vi "WHD_VEten_0.1.1_WS_BIDIR.vi"() -> ()   [LabVIEW 2015]
uses:
  <vilib>/NI_Real-Time Target Support.lvlib
  <vilib>/rvi/interface/nirviReadWriteControl/nirviReadWriteControl.xnode
  <vilib>/rvi/interface/nirviMethod/nirviMethod.xnode
  <vilib>/rvi/interface/nirviOpenFPGA/nirviOpenFPGA.xnode
  <vilib>/rvi/interface/nirviCloseFPGA/nirviCloseFPGA.xnode
  <vilib>/userdefined/High Color/nirio_resource_hc.ctl
  <vilib>/rvi/errors/niLvFpgaMergeErrorWithErrorCode.vi
  <vilib>/Utility/file.llb/Write Delimited Spreadsheet (string).vi
  <vilib>/RTwatchdog.llb/Watchdog expiration actions.ctl
  <vilib>/nisyscfg/nisyscfg.lvlib
  AURA_Wheel/Json2Labv.lvlib
  AURA_Wheel/AuraWheelAPI/AuraWheel.lvlib
  <vilib>/rvi/errors/niLvFpgaAdjustHostInterfaceError.vi
  NiFpgaLv.dll
  <vilib>/Utility/error.llb/Error Cluster From Error Code.vi
  <vilib>/LabVIEW Targets/FPGA/cRIO/shared/nicrio_ModuleControls/nicrio_cRIO-9234_DataRatesRing2.ctl
  <vilib>/FPGAPlugInAG/cRIO-9031/niLvFpga_Run_cRIO-9031.vi
  <vilib>/FPGAPlugInAG/cRIO-9031/niLvFpga_Reset_cRIO-9031.vi
  FPGA Bitfiles/W&RDArabia_FPGATarget_FPGA8a2wsBIdirec_yJvL9yuTbZw.lvbitx
  <vilib>/FPGAPlugInAG/cRIO-9031/niLvFpga_Open_cRIO-9031.vi
  <vilib>/FPGAPlugInAG/cRIO-9031/niLvFpga_ConfigureFifo_cRIO-9031.vi
  <vilib>/FPGAPlugInAG/cRIO-9031/niLvFpga_StartFifo_cRIO-9031.vi
  <vilib>/FPGAPlugInAG/cRIO-9031/niLvFpga_ReadFifo_cRIO-9031.vi
  <vilib>/FPGAPlugInAG/cRIO-9031/niLvFpga_StopFifo_cRIO-9031.vi
  <vilib>/FPGAPlugInAG/cRIO-9031/niLvFpga_Close_cRIO-9031.vi
panel:
  in  "Digital?":bool=TRUE
  out "Direction 0?":bool
  out "Boton Adquirir?":bool
  out "Wheel detected2?":bool=TRUE
  out "Wheel detected1?":bool=TRUE
  in  "Timeout ruedas":dbl
  in  "Borrar archivos\nadquisicion con error":bool
  in  "Able watchdog?":bool
  in  "Reset watchdog?":bool
  in  "Leer config RFID NEM":bool
  in  "bytes to read":i32
  in  "DeviceAddress":u8
  in  "timeout ms (60000)":i32
  in  "Max archivos":u32=2
  in  "Bytes libre despues de borrar":u32=2
  in  "Bytes min libre":u32=2
  in  "Nº de acelerómetros":i32
  in  "Nº inductivos":i32
  in  "Offset_rueda WS 1":fxp<+/-,24,-4>=0.004999998956918716 format="%.27g"
  out "TAGs_AURAwheel":string[][](array[string])
  out "Plataformas?":bool
  out "Nº Ejes":i32[](array[numeric])
  out "Nº UTs":i32
  out "it-read-LR6":i32[](array[numeric])
  out "it-LR6":i32
  out "RFID_LR6_Error":errorcluster
  out "Series_flota":string[](array[string])
  out "Tabla_flota":string[][](array[string])
  out "Puntos medios de las ventanas":dbl[][](array[numeric])
  out "configuration file path":path=path "c:/Parametros.cfg"
  in  "IP synchr":string
  out "data":cluster{"status":string}
  out "confRFID":path=path "c:/RFID/TAGS.csv"
  out "TAGS leidos":path=path "c:/RFID/TAGS.csv"
  in  "Use Aura?":bool
  in  "Parametros AuraWheel":string[](array[string])
  in  "Parámetros acelerómetros":dbl[](array[numeric])
  in  "Acquisition time":dbl=10.0
  in  "Acquire":bool
  out "Fin":bool
  out "Contador":i32=1
  out "Path TEST":path=path "c:/TEST"
  out "Fallo fotocelula":bool
  out "Path_Borrar":path=path "c:/Trenes"
  out "Longitud de la unidad":dbl
  out "Aviso no detección":string
  out "Time to Acquire Block (ms)":i32
  out "Distancia de acelerómetros":dbl[](array[numeric])
  out "Block Size":u32
  out "Distancias generales":dbl[](array[numeric])
  in  "Reset del controlador":bool
  in  "Configuración":bool
  in  "Parar la aplicación":bool
  out "RFID":bool=TRUE
  out "date/time string":string
  out "Timeout ruedas":bool
  out "Tiempo":dbl
  out "Inicio pasada":timestamp
  out "Ultimo TEST":timestamp
  out "Power Supply":bool=TRUE
  out "Status":string
  out "RFID_ID":refnum<k5>
  out "DC OK":string
  out "Aviso temperatura":string
  in  "Tab Control":T1(tab)=enum."Parameters"
  out "V (m/s)":dbl
  out "Temperature (ºC)":dbl
  out "Max Wheel RMS":dbl[][](array[numeric])
  out "result":bool
  out "TAGs":string[](array[string])
  out "Parar":bool
  out "TAGs LR6":string[](array[string])
  out "TAGs HEX":string[](array[string])
  out "Digital wheels":sgl[](graph)
  out "Current Wheel sensor":sgl[][](graph)
  out "File Name":path[](array[path])
  out "Train pass time (s)":dbl
  out "Acquisition extra time (s)":dbl
  out "Detected axles":i32
  out "Buffer Underflow":bool
  out "Buffer Overflow":bool
  out "Hard drive status (bytes)":i64
  out "created path":path
  out "Nº Wheel 1":i32
  out "Nº Wheel 2":i32
  out "Train axles":i32
  out "Valid \nfile?":bool
  in  "AURA wheel test":bool
  out "T fuera rango":bool
  in  "Frecuency rate (Hz)":dbl=25600.0
  in  "Samples per channel FIFO":u32=5000
  in  "Extra time detection (s)":dbl=1.0
  in  "dt RMS":dbl=256.0
  in  "Frecuency rate and CRIO module":T2=2 items=["51.200 kS/s (NI 9234)"=1, "25.600 kS/s (NI 9234)"=2, "17.067 kS/s (NI 9234)"=3, "12.800 kS/s (NI 9234)"=4, "10.240 kS/s (NI 9234)"=5, "8.533 kS/s (NI 9234)"=6, "7.314 kS/s (NI 9234)"=7, "6.400 kS/s (NI 9234)"=8, "5.689 kS/s (NI 9234)"=9, "5.120 kS/s (NI 9234)"=10, "4.654 kS/s (NI 9234)"=11, "4.267 kS/s (NI 9234)"=12, "3.938 kS/s (NI 9234)"=13, "3.657 kS/s (NI 9234)"=14, "3.413 kS/s (NI 9234)"=15, "3.200 kS/s (NI 9234)"=16, "3.012 kS/s (NI 9234)"=17, "2.845 kS/s (NI 9234)"=18, "2.695 kS/s (NI 9234)"=19, "2.560 kS/s (NI 9234)"=20, "2.438 kS/s (NI 9234)"=21, "2.328 kS/s (NI 9234)"=22, "2.226 kS/s (NI 9234)"=23, "2.133 kS/s (NI 9234)"=24, "2.048 kS/s (NI 9234)"=25, "1.969 kS/s (NI 9234)"=26, "1.896 kS/s (NI 9234)"=27, "1.829 kS/s (NI 9234)"=28, "1.765 kS/s (NI 9234)"=29, "1.707 kS/s (NI 9234)"=30, "1.652 kS/s (NI 9234)"=31]
  in  "RFID Port":u16=2189
  in  "RFID IP":string="192.168.106.99"
  in  "Offset_rueda WS 2":fxp<+/-,24,-4>=0.004999998956918716 format="%.27g"
  in  "Count(mSec)":u32=2
  in  "LR6 IP address":string="192.168.106.94"
  in  "Port LR6":u16=2001
  in  "RFID NEM on?":bool
  in  "RFID LR6 on?":bool
  in  "Zero channel WS1?":bool
  in  "Zero channel WS2?":bool
  out "Parameters":bool=TRUE
  out "Distances of the system":bool=TRUE
  out "RFID Error":errorcluster
  out "FPGA error":errorcluster
  out "Write/read error":errorcluster
  out "Units and axles":bool=TRUE
  out "RFID":bool=TRUE
  out "AURA error":errorcluster
  out "Response headers":string
  out "Numeric 3":i32
  out "Loop":i32
  out "Watchdog config":T3={"reset system"=FALSE, "restart LabVIEW Runtime"=FALSE, "occurrence"=FALSE, "trigger protocol"=enum."active high", "trigger line"=enum."none", "disable watchdog on VI exit"=TRUE}
  # "Last train detected"
  # "Error!!"
  # "Memory status"
  # "Samples parameters"
  # "Acquisition parameters"
  # "Other parameters"
  # "Configuration data load"
  # "Errores!!"
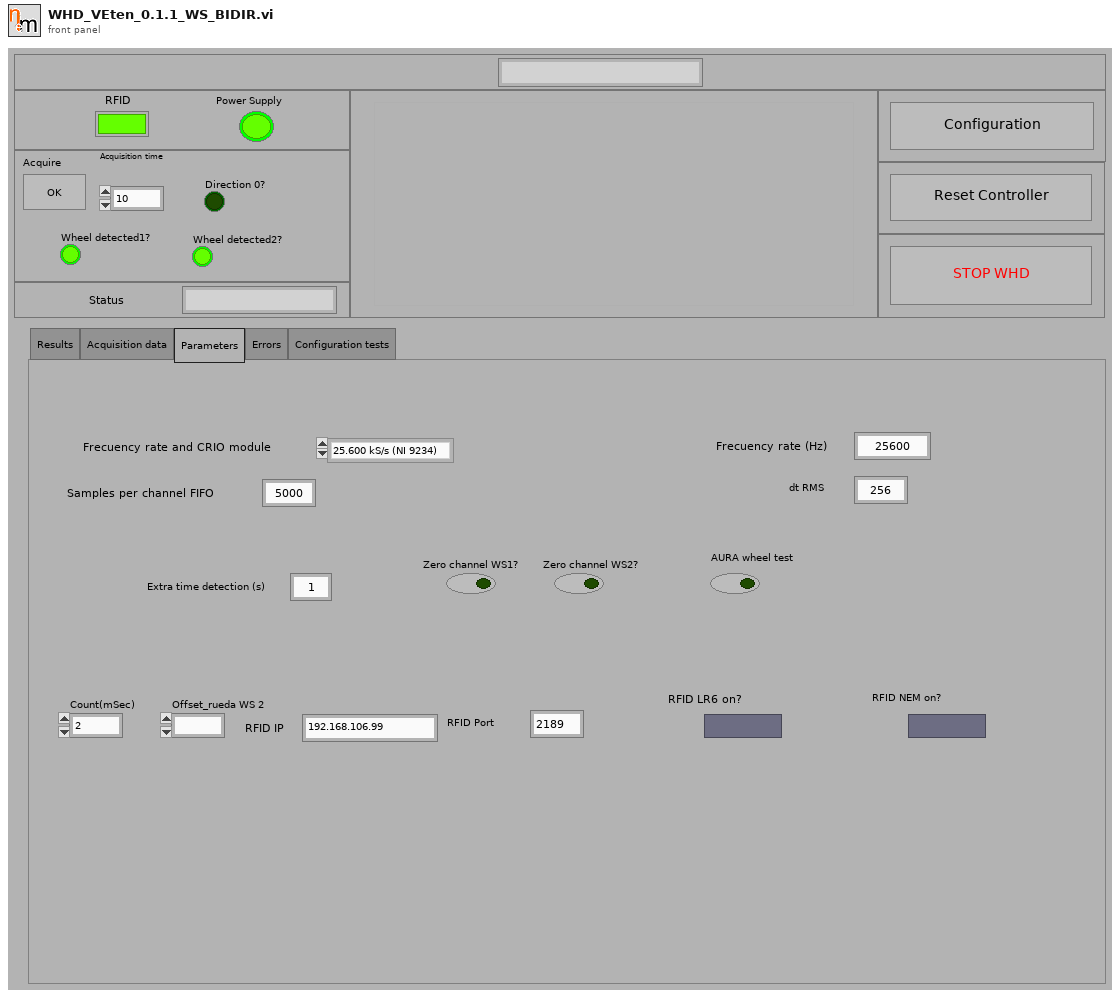
[diagram p1: front panel]
types:
  T1 = enum32{"Results", "Acquisition data", "Parameters", "Errors", "Configuration tests"}
  T2 = typedef "nicrio_cRIO-9234_DataRatesRing2.ctl" = u8
  T3 = typedef "Watchdog expiration actions.ctl" = cluster{"reset system":bool, "restart LabVIEW Runtime":bool, "occurrence":bool, "trigger protocol":enum16{"active high", "active low", "open collector"}, "trigger line":enum16{"none", "line 0", "line 1", "line 2", "line 3", "line 4", "line 5", "line 6", "line 7", "SMB line 0"}, "disable watchdog on VI exit":bool}
  T4 = typedef "nirio_resource_hc.ctl" = tag
  T5 = enum16{"Standard", "Buffered", "CRLF", "Immediate"}
  T6 = enum16{"open", "replace", "create", "open or create", "replace or create", "replace or create with confirmation"}
  T7 = enum16{"big-endian, network order", "native, host order", "little-endian"}
  T8 = cluster{"error IO":errorcluster, bool[], u32[], string[], dbl[]}
  T9 = cluster{"g_ts":dbl, "p_sp":dbl, "p_tp":dbl, "p_tg":cluster{"tg_n":dbl, "tg_t":string}[], "p_ax":cluster{"ax_n":dbl, "ax_sp":dbl, "ax_wh":cluster{"wh_p":dbl, "wh_a1":dbl, "wh_a2":dbl, "wh_a3":dbl, "wh_a4":dbl}[]}[]}
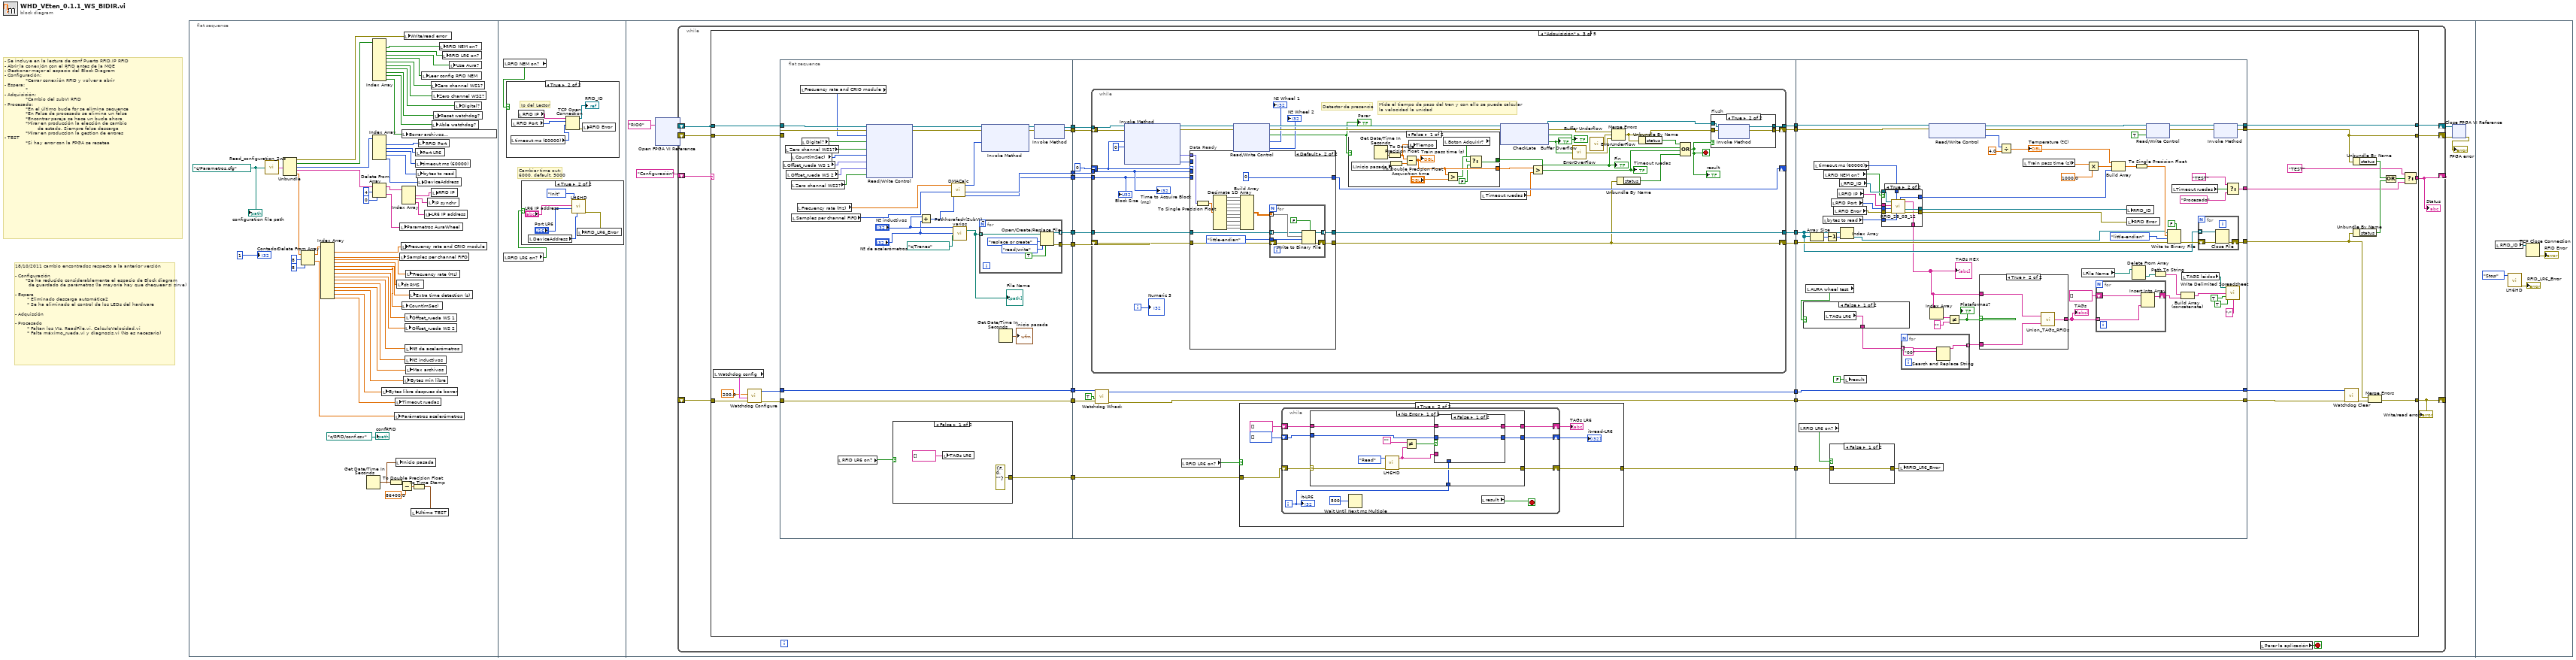
[diagram p0: block diagram]
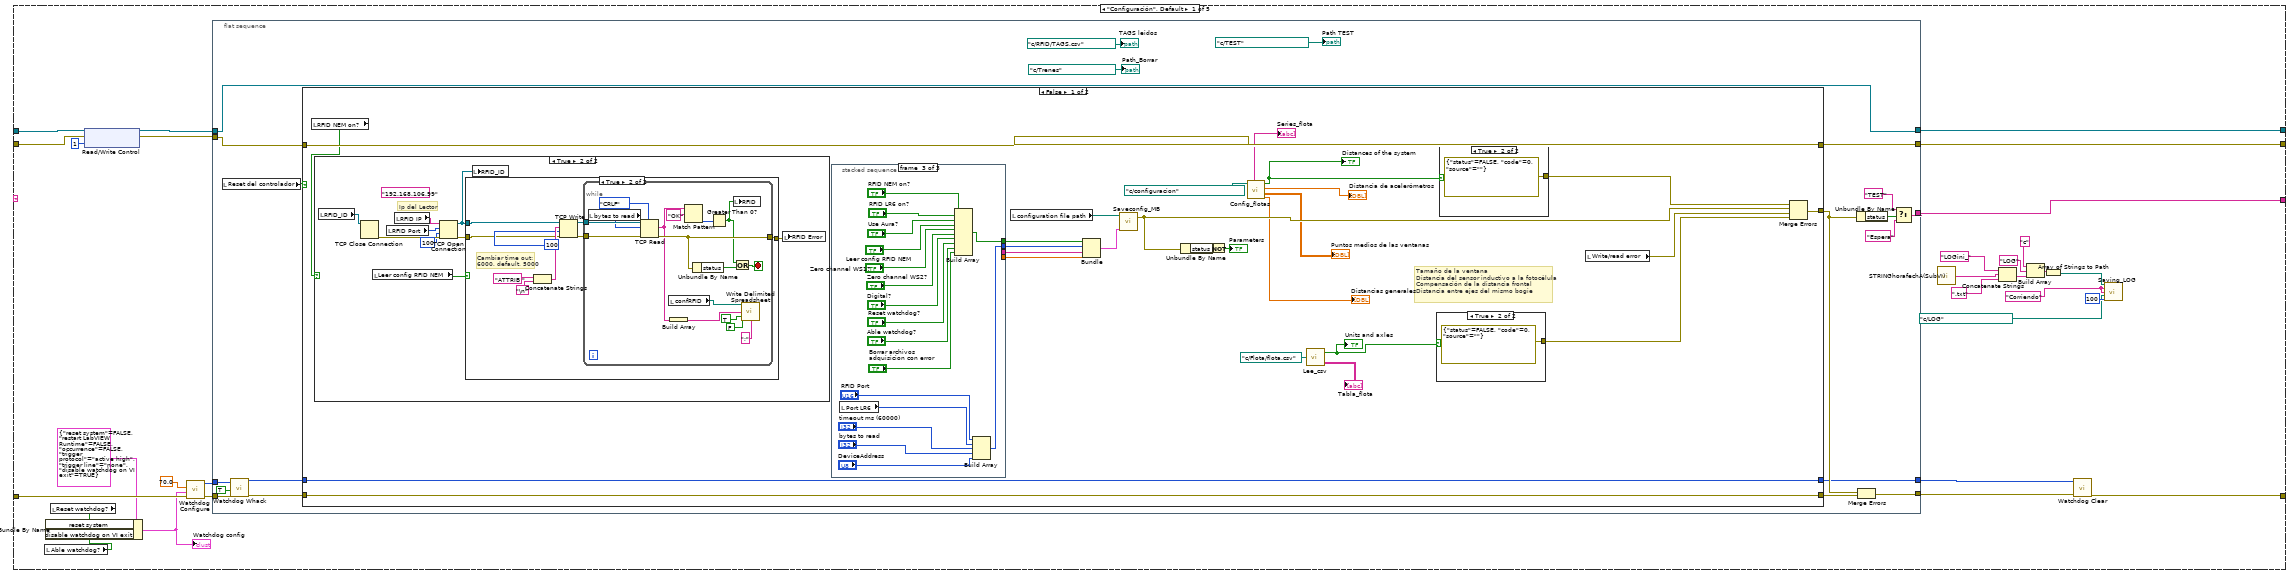
[diagram p4: hidden frame]
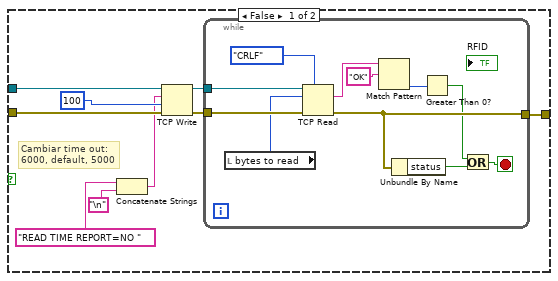
[diagram p6: hidden frame]
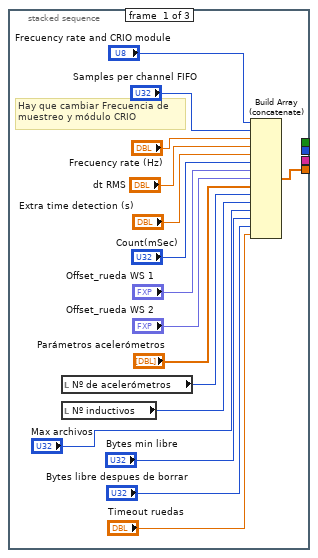
[diagram p7: hidden frame]
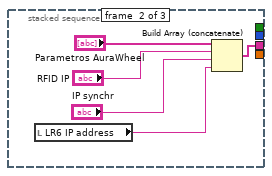
[diagram p8: hidden frame]
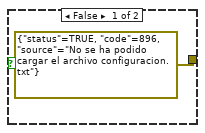
[diagram p9: hidden frame]
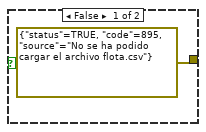
[diagram p10: hidden frame]
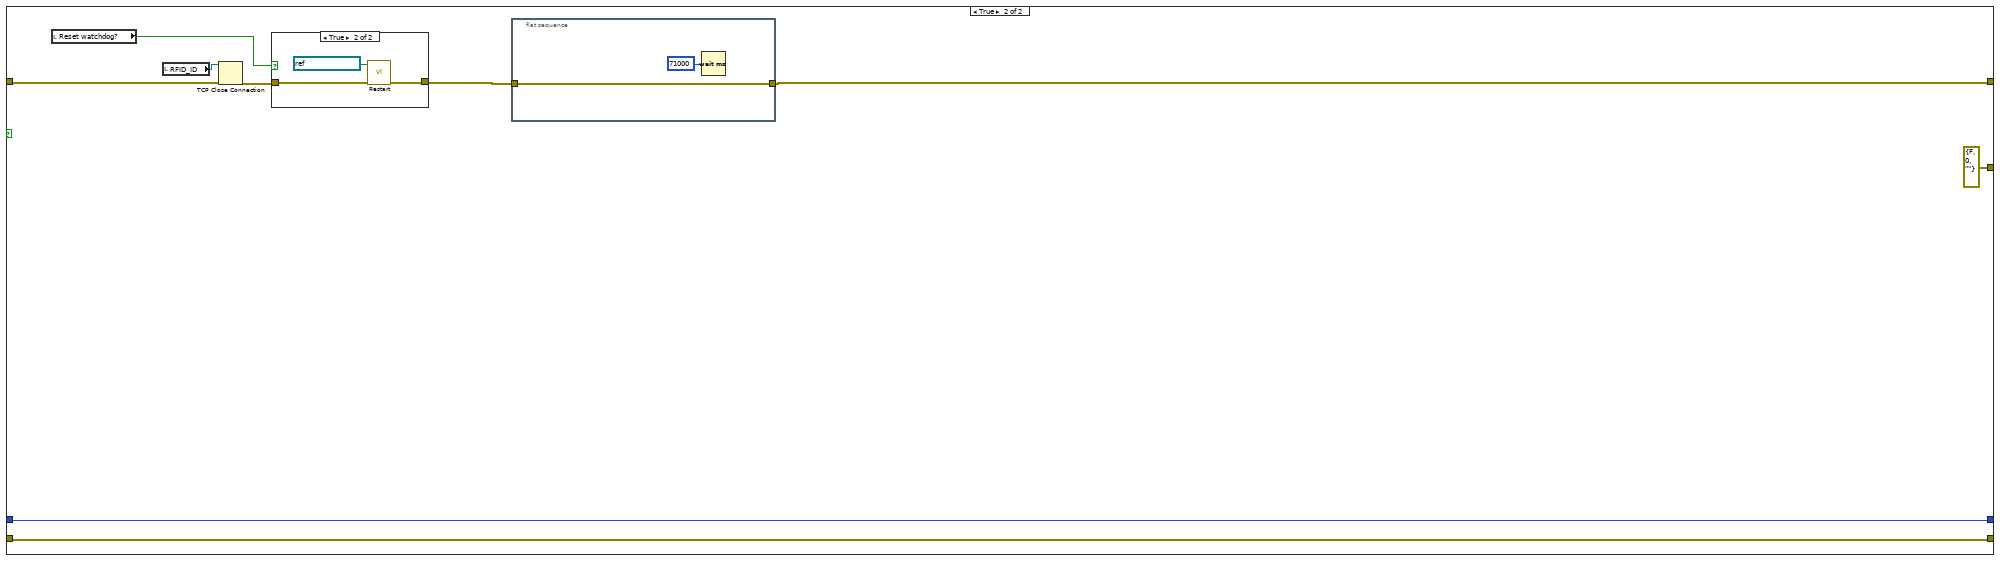
[diagram p11: hidden frame]
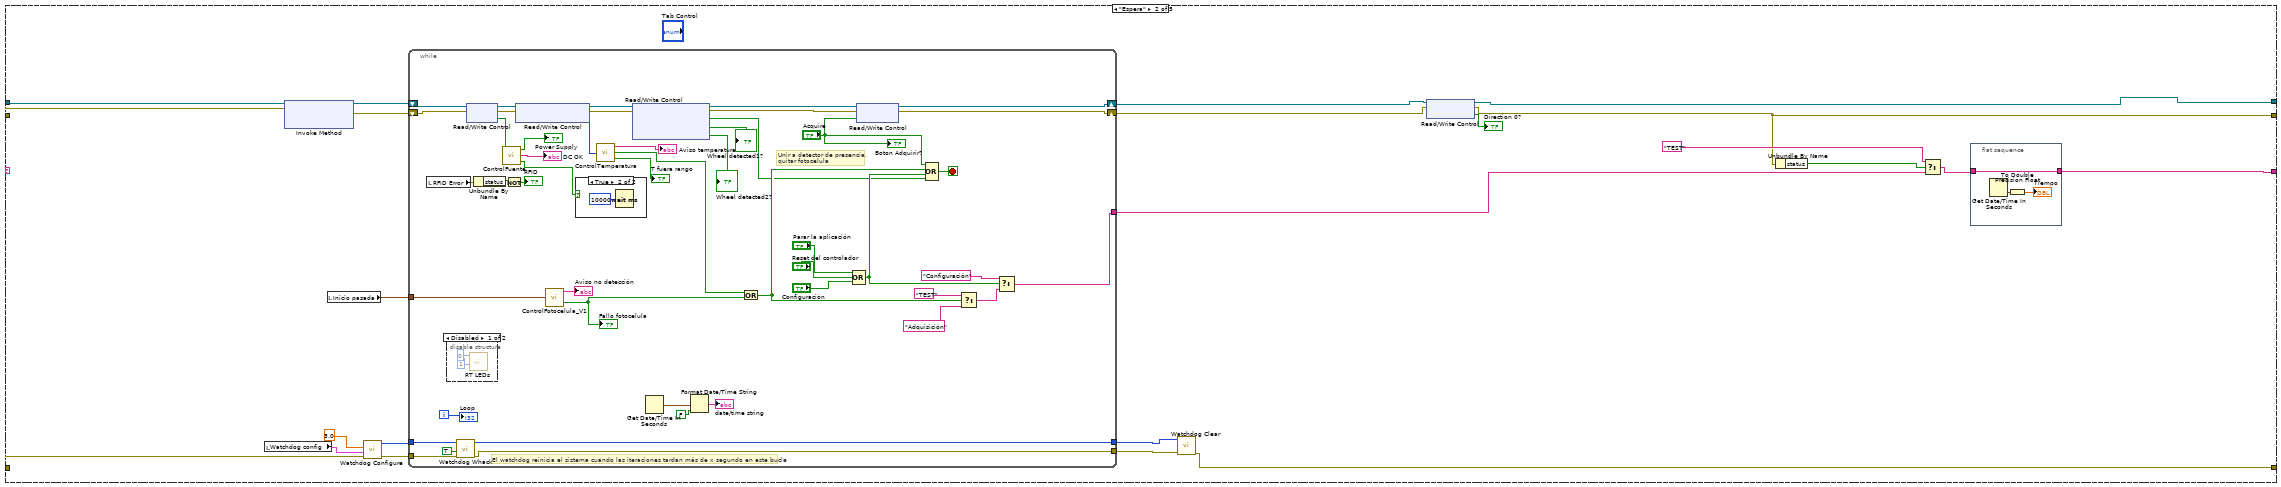
[diagram p13: hidden frame]
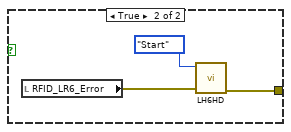
[diagram p16: hidden frame]
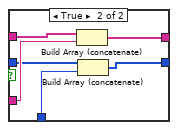
[diagram p18: hidden frame]
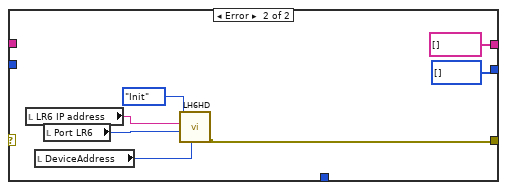
[diagram p19: hidden frame]
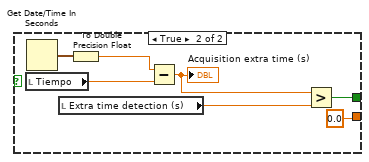
[diagram p20: hidden frame]
diagram:
  # "18/10/2011 cambio encontrados respecto a la anterior versión\n\n- Configuración\n       *Se ha reducido considerablemente el espacio de Block diagram\n         de guardado de parámetros (la mayoría hay que chequear si sirve)\n\n- Espera\n        * Eliminado descarga automática2\n        * Se ha eliminado el control de los LEDs del hardware\n       \n- Adquisción\n\n- Procesado\n        * Faltan los VIs, ReadFile.vi, CalculoVelocidad.vi\n        * Falta máximo_rueda.vi y diagnosis.vi (No es necesario)"
  # "- Se incluye en la lectura de conf Puerto RFID,IP RFID\n- Abrir la conexión con el RFID antes de la MQE\n- Gestionar mejor el espacio del Block Diagram\n- Configuración:\n              *Cerrar conexión RFID y volver a abrir\n- Espera:\n              *\n- Adquisición:\n              *Cambio del subVI RFID\n- Procesado:\n              *En el último bucle for se elimina sequence\n              *En False de procesado se elimina un false\n              *Encontrar pareja se hace un bucle ahora\n              *Mirar en producción la elección de cambio\n                      de estado. Siempre false descarga \n              *Mirar en produccion la gestion de errores\n- TEST\n              *Si hay error con la FPGA se resetea"
  n1 = flat-sequence {
    frame #0 {
      w38 = path "c:/Parametros.cfg" ("configuration file path")
      n2 = call "Read_configuration_2ws.vi"("configuration file path"=w38) -> ("output cluster"=w37:T8)
      n3 = Unbundle(w37) -> ("error IO"=w42:errorcluster, w41:bool[], w40:u32[], w29:string[], w35:dbl[])
      n4 = Delete From Array(array=w35, length=8, index=8) -> (deleted portion=w31:dbl[], array with subset deleted=w34:dbl[])
      n5 = Index Array(array=w34) -> (element #1=w49:dbl, element #2=w48:dbl, element #3=w47:dbl, element #4=w46:dbl, element #5=w45:dbl, element #6=w19:dbl, element #7=w18:dbl, element #8=w1:dbl, element #9=w17:dbl, element #10=w16:dbl, element #11=w15:dbl, element #12=w14:dbl, element #13=w13:dbl, element #14=w2:dbl)  [unwired: 14 in]
      n6 = Get Date/Time In Seconds() -> (seconds since 1Jan1904=w51:timestamp)
      n7 = Index Array(array=w41) -> (element #1=w44:bool, element #2=w43:bool, element #3=w30:bool, element #4=w9:bool, element #5=w8:bool, element #6=w7:bool, element #7=w6:bool, element #8=w5:bool, element #9=w4:bool, element #10=w3:bool)  [unwired: 10 in]
      n8 = Index Array(array=w40) -> (element #1=w36:u32, element #2=w20:u32, element #3=w12:u32, element #4=w11:u32, element #5=w10:u32)  [unwired: 5 in]
      n9 = Delete From Array(array=w29, length=4, index=0) -> (deleted portion=w23:string[], array with subset deleted=w28:string[])
      n10 = local write "Bytes libre despues de borrar"(w13) -> ()
      n11 = To Double Precision Float(number=w51) -> (double precision float=w53:dbl)
      n12 = local write "Parámetros acelerómetros"(w31) -> ()
      n13 = local write "Timeout ruedas"(w2) -> ()
      n14 = local write "Inicio pasada"(w51) -> ()
      n15 = local write "dt RMS"(w46) -> ()
      n16 = local write "Samples per channel FIFO"(w48) -> ()
      n17 = local write "Parametros AuraWheel"(w23) -> ()
      n18 = Subtract(x=w53, y=86400.0) -> (x-y=w52:dbl)
      n19 = local write "Frecuency rate and CRIO module"(w49) -> ()
      n20 = local write "Borrar archivos\nadquisicion con error"(w3) -> ()
      n21 = Index Array(array=w28) -> (element #1=w22:string, element #2=w24:string, element #3=w21:string)  [unwired: 3 in]
      n22 = local write "Count(mSec)"(w19) -> ()
      n23 = local write "Bytes min libre"(w14) -> ()
      n24 = local write "Write/read error"(w42) -> ()
      n25 = local write "Offset_rueda WS 2"(w1) -> ()
      n26 = local write "Offset_rueda WS 1"(w18) -> ()
      n27 = local write "Nº de acelerómetros"(w17) -> ()
      n28 = local write "Nº inductivos"(w16) -> ()
      n29 = local write "Frecuency rate (Hz)"(w47) -> ()
      n30 = local write "Max archivos"(w15) -> ()
      n31 = local write "Extra time detection (s)"(w45) -> ()
      n32 = To Time Stamp(1:w52) -> (0:w50:timestamp)
      n33 = local write "Ultimo TEST"(w50) -> ()
      n34 = local write "Port LR6"(w20) -> ()
      n35 = local write "timeout ms (60000)"(w12) -> ()
      n36 = local write "bytes to read"(w11) -> ()
      n37 = local write "DeviceAddress"(w10) -> ()
      n38 = local write "RFID Port"(w36) -> ()
      n39 = local write "Leer config RFID NEM"(w9) -> ()
      n40 = local write "LR6 IP address"(w21) -> ()
      n41 = local write "IP synchr"(w24) -> ()
      n42 = local write "Zero channel WS1?"(w8) -> ()
      n43 = local write "RFID IP"(w22) -> ()
      n44 = local write "Able watchdog?"(w4) -> ()
      n45 = local write "Zero channel WS2?"(w7) -> ()
      n46 = local write "Reset watchdog?"(w5) -> ()
      n47 = local write "RFID NEM on?"(w44) -> ()
      n48 = local write "RFID LR6 on?"(w43) -> ()
      n49 = local write "Use Aura?"(w30) -> ()
      n50 = local write "Digital?"(w6) -> ()
      "Contador" <- 1
      "confRFID" <- path "c:/RFID/conf.csv" ("file path (use dialog)")
      "configuration file path" <- w38
    }
    frame #1 {
      # "Cambiar time out:\n6000, default, 5000"
      n51 = local read "RFID NEM on?"() -> (w56:bool)
      n52 = local read "RFID LR6 on?"() -> (w55:bool)
      n53 = case shown="True" w56 {
        frame False {
        }
        frame True {
          # "Ip del Lector"
          n54 = local read "timeout ms (60000)"() -> (w62:i32)
          n55 = local read "RFID Port"() -> (w64:u16)
          n56 = local read "RFID IP"() -> (w65:string)
          n57 = TCP Open Connection(address=w65, remote port or service name=w64, timeout ms (60000)=w62) -> (connection ID=→"RFID_ID":refnum<k5>, error out=w63:errorcluster)  [unwired: 1 in, 1 out]
          n58 = local write "RFID Error"(w63) -> ()
        }
      }
      n59 = case shown="True" w55 {
        frame False {
        }
        frame True {
          n60 = local read "DeviceAddress"() -> (w57:u8)
          n61 = call "LH6HD.vi"("DeviceAddress"=w57, "Reader Port"="Port LR6", "IP Address"="LR6 IP address", "Action"=enum16{"Init", "Start", "Read", "Stop", "Exit"}."Init") -> ("error out"=w61:errorcluster)  [unwired: 6 in, 1 out]
          n62 = local write "RFID_LR6_Error"(w61) -> ()
        }
      }
    }
    frame #2 {
      n63 = xnode "Open FPGA VI Reference"("resource name"=T4 "RIO0") -> ("FPGA VI Reference Out"=w73:refnum<k20>, "error out"=w72:errorcluster)  [unwired: 1 in]
      n64 = while {
        shift-right: [w77] -> _
        shift-left: "Configuración" -> [w82]
        shift-right: [w75] -> w69
        shift-left: w73 -> [w81]
        shift-right: [w74] -> w68
        shift-left: w72 -> [w80]
        shift-right: [w79] -> _
        shift-left: _ -> [w78]
        stop <- w76 stop-if-true
        n65 = case shown="\"Adquisición\"" w82 {
          tunnel: [w111 w283 w360 w695 w942] -> w77
          tunnel: [w110 w271 w374 w703 w941] -> w75
          tunnel: [w112 w270 w375 w690 w939] -> w74
          tunnel: w81 -> [w99 w288 w382 w703 w941]
          tunnel: w80 -> [w97 w286 w381 w690 w940]
          tunnel: [w103 w277 w372 w693 w929] -> w79
          tunnel: w78 -> [w109 w282 w356 w689 w934]
          frame "Configuración", Default {
            w83 = "Corriendo" ("Report")
            n66 = local read "Able watchdog?"() -> (w94:bool)
            n67 = local read "Reset watchdog?"() -> (w101:bool)
            n68 = Bundle By Name(cluster=T3 {"reset system"=FALSE, "restart LabVIEW Runtime"=FALSE, "occurrence"=FALSE, "trigger protocol"=enum."active high", "trigger line"=enum."none", "disable watchdog on VI exit"=TRUE} ("expiration actions"), "reset system"=w101, "disable watchdog on VI exit"=w94) -> (w100:T3)
            "Watchdog config" <- w100
            n69 = xnode "Read/Write Control"("FPGA VI Reference In"=w99, "error in"=w97, "Cycles to Filter"=u16 1) -> ("FPGA VI Reference Out"=w98:refnum<k20>, "error out"=w96:errorcluster)
            n70 = call <vilib>:"Watchdog Configure.vi"("error in (no error)"=w109, "expiration actions"=w100, "timeout (1 sec)"=70.0) -> ("error out"=w106:errorcluster, "watchdogID"=w107:u64)  [unwired: 1 in, 2 out]
            n71 = flat-sequence {
              tunnel: [w123] -> w112
              tunnel: [w131] -> w111
              tunnel: w98 -> [w124]
              tunnel: [w124] -> w110
              tunnel: [w126] -> w104
              tunnel: w96 -> [w121]
              tunnel: w107 -> [w119]
              tunnel: w106 -> [w118]
              tunnel: [w116] -> w105
              frame #0 {
                n72 = local read "Reset del controlador"() -> (w120:bool)
                n73 = call <vilib>:"Watchdog Whack.vi"("error in (no error)"=w118, "reset watchdog after expire? (F)"=TRUE, "watchdogID in"=w119) -> ("error out"=w114:errorcluster, "watchdogID out"=w115:u64)  [unwired: 2 in, 1 out]
                n74 = case shown="False" w120 {
                  tunnel: w121 -> [w158 w261]
                  tunnel: [w158 w260] -> w123
                  tunnel: [w144 errorcluster {"status"=FALSE, "code"=0, "source"=""} ("error IO")] -> w122
                  tunnel: [w136 w259] -> w116
                  tunnel: w115 -> [w136 w259]
                  tunnel: w114 -> [w135 w258]
                  tunnel: [w135 w258] -> w113
                  frame False {
                    # "Tamaño de la ventana\nDistancia del sensor inductivo a la fotocélula\nCompensación de la distancia frontal\nDistancia entre ejes del mismo bogie"
                    n75 = local read "RFID NEM on?"() -> (w134:bool)
                    n76 = case shown="True" w134 {
                      frame False {
                      }
                      frame True {
                        (unwired) "192.168.106.99" ("address")
                        # "Ip del Lector"
                        n77 = local read "RFID_ID"() -> (w166:refnum<k5>)
                        n78 = TCP Close Connection(connection ID=w166) -> (error out=w167:errorcluster)  [unwired: 2 in, 1 out]
                        n79 = local read "Leer config RFID NEM"() -> (w159:bool)
                        n80 = local read "RFID Port"() -> (w164:u16)
                        n81 = local read "RFID IP"() -> (w163:string)
                        n82 = TCP Open Connection(address=w163, remote port or service name=w164, timeout ms (60000)=100, error in (no error)=w167) -> (connection ID=w165:refnum<k5>, error out=w160:errorcluster)  [unwired: 1 out]
                        n83 = case shown="True" w159 {
                          tunnel: w165 -> [w176 w190]
                          tunnel: [w174 w188] -> w161
                          tunnel: w160 -> [w171 w189]
                          frame False {
                            # "Cambiar time out:\n6000, default, 5000"
                            n84 = Concatenate Strings("READ TIME REPORT=NO " ("data in"), "\n") -> (w168:string)
                            n85 = TCP Write(connection ID=w176, data in=w168, error in (no error)=w171, 9:100 ("timeout ms (25000)")) -> (connection ID out=w172:refnum<k5>, error out=w173:errorcluster)  [unwired: 1 out]
                            n86 = while {
                              tunnel: w173 -> [w186]
                              tunnel: w172 -> [w185]
                              tunnel: [w184] -> w174
                              stop <- w181 stop-if-true
                              n87 = local read "bytes to read"() -> (w177:i32)
                              n88 = TCP Read(connection ID=w185, bytes to read=w177, error in (no error)=w186, 7:T5."CRLF" ("mode (standard)")) -> (data out=w179:string, error out=w184:errorcluster)  [unwired: 1 in, 1 out]
                              n89 = Match Pattern(string=w179, regular expression="OK") -> (offset past match=w182:i32)  [unwired: 4 out]
                              n90 = Unbundle By Name(w184) -> ("status"=w180:bool)
                              n91 = Greater Than 0?(x=w182) -> (x > 0?=w178:bool)
                              n92 = Or(x=w178, y=w180) -> (x .or. y?=w181:bool)
                            }
                          }
                          frame True {
                            # "Cambiar time out:\n6000, default, 5000"
                            n93 = Concatenate Strings("ATTRIB " ("data in"), "\n") -> (w196:string)
                            n94 = TCP Write(connection ID=w190, data in=w196, error in (no error)=w189, 9:100 ("timeout ms (25000)")) -> (connection ID out=w193:refnum<k5>, error out=w192:errorcluster)  [unwired: 1 out]
                            n95 = while {
                              tunnel: w192 -> [w211]
                              tunnel: w193 -> [w210]
                              tunnel: [w209] -> w188
                              stop <- w206 stop-if-true
                              n96 = local read "bytes to read"() -> (w198:i32)
                              n97 = TCP Read(connection ID=w210, bytes to read=w198, error in (no error)=w211, 7:T5."CRLF" ("mode (standard)")) -> (data out=w201:string, error out=w209:errorcluster)  [unwired: 1 in, 1 out]
                              n98 = local read "confRFID"() -> (w200:path)
                              n99 = Build Array(w201) -> (w199:string[])
                              n100 = Match Pattern(string=w201, regular expression="OK") -> (offset past match=w207:i32)  [unwired: 4 out]
                              n101 = Unbundle By Name(w209) -> ("status"=w205:bool)
                              n102 = Greater Than 0?(x=w207) -> (x > 0?=w197:bool)
                              n103 = local write "RFID"(w197) -> ()
                              n104 = Or(x=w197, y=w205) -> (x .or. y?=w206:bool)
                              n105 = call-poly <vilib>:"Write Delimited Spreadsheet.vi"("file path (dialog if empty)"=w200, "1D data"=w199, "append to file? (new file:F)"=FALSE ("transpose? (no:F)"), "transpose? (no:F)"=TRUE ("append to file? (new file:F)"), "delimiter (\\t)"=";" ("delimiter (\\t)")) -> ()  [unwired: 9 in, 2 out]
                            }
                          }
                        }
                        n106 = local write "RFID_ID"(w165) -> ()
                        n107 = local write "RFID Error"(w161) -> ()
                      }
                    }
                    n108 = stacked-sequence {
                      tunnel: [w224 _ _] -> w148
                      tunnel: [_ w233 _] -> w147
                      tunnel: [_ _ w247] -> w149
                      tunnel: [_ _ w246] -> w150
                      frame #0 {
                        # "Hay que cambiar Frecuencia de\nmuestreo y módulo CRIO"
                        n109 = local read "Nº de acelerómetros"() -> (w218:i32)
                        n110 = local read "Nº inductivos"() -> (w217:i32)
                        n111 = Build Array (concatenate)("Frecuency rate and CRIO module", "Samples per channel FIFO", "Frecuency rate (Hz)", "dt RMS", "Extra time detection (s)", "Count(mSec)", "Offset_rueda WS 1", "Offset_rueda WS 2", "Parámetros acelerómetros", w218, w217, "Max archivos", "Bytes min libre", "Bytes libre despues de borrar", "Timeout ruedas") -> (w224:dbl[])
                      }
                      frame #1 {
                        n112 = local read "LR6 IP address"() -> (w229:string)
                        n113 = Build Array (concatenate)("Parametros AuraWheel", "RFID IP", "IP synchr", w229) -> (w233:string[])
                      }
                      frame #2 {
                        n114 = local read "Port LR6"() -> (w243:u16)
                        n115 = Build Array("RFID NEM on?", "RFID LR6 on?", "Use Aura?", "Leer config RFID NEM", "Zero channel WS1?", "Zero channel WS2?", "Digital?", "Reset watchdog?", "Able watchdog?", "Borrar archivos\nadquisicion con error") -> (w246:bool[])
                        n116 = Build Array("RFID Port", w243, "timeout ms (60000)", "bytes to read", "DeviceAddress") -> (w247:i32[])
                      }
                    }
                    n117 = local read "configuration file path"() -> (w145:path)
                    n118 = Bundle(w150, w149, w147, w148) -> (w146:cluster{bool[], i32[], string[], dbl[]})  [unwired: 1 in]
                    n119 = call "Saveconfig_MB.vi"("configuration file path"=w145, "Configuracion"=w146) -> ("error out"=w153:errorcluster)  [unwired: 4 in]
                    n120 = Unbundle By Name(w153) -> ("status"=w154:bool)
                    n121 = Not(x=w154) -> (.not. x?=→"Parameters":bool)
                    n122 = call "Config_flotas.vi"("file path (dialog if empty)"=path "c:/configuracion") -> ("Distancias generales"=→"Distancias generales":dbl[], "Puntos medios de las ventanas"=→"Puntos medios de las ventanas":dbl[][], "Distancia de acelerómetros"=→"Distancia de acelerómetros":dbl[], "Distacias y medidas de dispositivos"=w143:bool, "Series_flota"=→"Series_flota":string[])  [unwired: 3 in]
                    "Distances of the system" <- w143
                    n123 = call "Lee_csv.vi"("Path"=path "c:/Flota/flota.csv") -> ("Tabla_flota"=→"Tabla_flota":string[][], "Lectura_OK?"=w140:bool)
                    "Units and axles" <- w140
                    n124 = case shown="True" w140 {
                      tunnel: [errorcluster {"status"=TRUE, "code"=895, "source"="No se ha podido cargar el archivo flota.csv"} ("error out") errorcluster {"status"=FALSE, "code"=0, "source"=""} ("error out")] -> w151
                      frame False {
                      }
                      frame True {
                      }
                    }
                    n125 = case shown="True" w143 {
                      tunnel: [errorcluster {"status"=TRUE, "code"=896, "source"="No se ha podido cargar el archivo configuracion.txt"} ("error out") errorcluster {"status"=FALSE, "code"=0, "source"=""} ("error out")] -> w156
                      frame False {
                      }
                      frame True {
                      }
                    }
                    n126 = local read "Write/read error"() -> (w152:errorcluster)
                    n127 = Merge Errors(w156, w153, w152, w151) -> (w144:errorcluster)
                  }
                  frame True {
                    n128 = local read "Reset watchdog?"() -> (w255:bool)
                    n129 = local read "RFID_ID"() -> (w263:refnum<k5>)
                    n130 = TCP Close Connection(connection ID=w263, error in (no error)=w261) -> (error out=w257:errorcluster)  [unwired: 2 out]
                    n131 = case shown="True" w255 {
                      tunnel: w257 -> [w264 w267]
                      tunnel: [w264 w266] -> w256
                      frame False {
                      }
                      frame True {
                        n132 = call <vilib>:"Restart.vi"("error in (no error)"=w267, "Session in"=refnum<k21> "localhost") -> ("error out"=w266:errorcluster)  [unwired: 7 in, 2 out]
                      }
                    }
                    n133 = flat-sequence {
                      tunnel: [w269] -> w260
                      tunnel: w256 -> [w269]
                      frame #0 {
                        n134 = Wait (ms)(milliseconds to wait=u32 71000) -> ()  [unwired: 1 out]
                      }
                    }
                  }
                }
                n135 = Unbundle By Name(w122) -> ("status"=w132:bool)
                n136 = Merge Errors(w122, w113) -> (w126:errorcluster)
                n137 = Select(t="TEST", s=w132, f="Espera") -> (s? t:f=w131:string)
                "Path_Borrar" <- path "c:/Trenes" ("file path (use dialog)")
                "Path TEST" <- path "c:/TEST" ("file path (use dialog)")
                "TAGS leidos" <- path "c:/RFID/TAGS.csv" ("file path (use dialog)")
              }
            }
            n138 = call "STRINGhorafechA(SubVI).vi"() -> ("STRINGhora_fecha"=w91:string)
            n139 = Concatenate Strings("LOGini_" ("string"), w91, ".txt" ("string")) -> (w93:string)
            n140 = Build Array("c", "LOG" ("element"), w93) -> (w90:string[])
            n141 = Array of Strings to Path(0:w90) -> (2:w86:path)  [unwired: 1 out]
            n142 = call <vilib>:"Watchdog Clear.vi"("error in (no error)"=w104, "watchdogID in"=w105) -> ("error out"=w103:errorcluster)  [unwired: 5 in]
            n143 = call "Saving_LOG.vi"("Path"=w86, "Report"=w83, "Report AURA"=w83, "Path Carpeta"=path "c:/LOG" ("file path (use dialog)"), "Nº Archivos Max"=100) -> ()  [unwired: 9 in, 2 out]
          }
          frame "Espera" {
            n144 = local read "Watchdog config"() -> (w276:T3)
            n145 = xnode "Invoke Method"("FPGA VI Reference In"=w288, "error in"=w286) -> ("FPGA VI Reference Out"=w287:refnum<k20>, "error out"=w285:errorcluster)  [unwired: 1 in]
            n146 = local read "Inicio pasada"() -> (w292:timestamp)
            n147 = call <vilib>:"Watchdog Configure.vi"("error in (no error)"=w282, "expiration actions"=w276, "timeout (1 sec)"=3.0) -> ("error out"=w281:errorcluster, "watchdogID"=w280:u64)  [unwired: 1 in, 2 out]
            n148 = while {
              tunnel: [w316] -> w291
              shift-right: [w306] -> w272
              shift-left: w287 -> [w318]
              shift-right: [w305] -> w273
              shift-left: w285 -> [w317]
              tunnel: w292 -> [w321]
              tunnel: w281 -> [w303]
              tunnel: w280 -> [w304]
              tunnel: [w302] -> w279
              tunnel: [w301] -> w278
              i -> [w299]
              stop <- w343 stop-if-true
              # "Unir a detector de presencia,\nquitar fotocelula"
              # "El watchdog reinicia el sistema cuando las iteraciones tardan más de x segundo en este bucle"
              n149 = local read "RFID Error"() -> (w324:errorcluster)
              n150 = disable-structure shown="Disabled" {
                frame Disabled {
                  n151 = call <vilib>:"RT LEDs.vi"("State"=1, "LED Num"=0) -> ()  [unwired: 1 in, 5 out]
                }
                frame Enabled {
                }
              }
              n152 = call <vilib>:"Watchdog Whack.vi"("error in (no error)"=w303, "reset watchdog after expire? (F)"=TRUE, "watchdogID in"=w304) -> ("error out"=w301:errorcluster, "watchdogID out"=w302:u64)  [unwired: 2 in, 1 out]
              n153 = xnode "Read/Write Control"("FPGA VI Reference In"=w318, "error in"=w317) -> ("FPGA VI Reference Out"=w334:refnum<k20>, "error out"=w333:errorcluster, "DC OK"=w338:bool)
              n154 = Unbundle By Name(w324) -> ("status"=w322:bool)
              n155 = call "ControlFuente.vi"("DC OK 3"=w338) -> ("DC OK 2"=→"Power Supply":bool, "DC OK"=→"DC OK":string, "Boolean"=w296:bool)
              n156 = Not(x=w322) -> (.not. x?=→"RFID":bool)
              n157 = xnode "Read/Write Control"("FPGA VI Reference In"=w334, "error in"=w333) -> ("FPGA VI Reference Out"=w330:refnum<k20>, "error out"=w329:errorcluster, "Chassis Temperature"=w336:i16)
              n158 = call "ControlFotocelula_V1.vi"("Tiempo de entrada a espera"=w321) -> ("Aviso no detección"=→"Aviso no detección":string, "Boolean"=w327:bool)
              "Fallo fotocelula" <- w327
              n159 = case shown="True" w296 {
                frame False {
                }
                frame True {
                  n160 = Wait (ms)(milliseconds to wait=u32 10000) -> ()  [unwired: 1 out]
                }
              }
              n161 = call "ControlTemperatura.vi"("Chassis Temperature"=w336) -> ("Aviso temperatura"=→"Aviso temperatura":string, "Boolean"=w297:bool, "T fuera rango"=→"T fuera rango":bool)
              n162 = xnode "Read/Write Control"("FPGA VI Reference In"=w330, "error in"=w329) -> ("FPGA VI Reference Out"=w320:refnum<k20>, "error out"=w319:errorcluster, "Detector de presencia"=w311:bool, "RuedaDetectada1?"=→"Wheel detected1?":bool, "RuedaDetectada2?"=→"Wheel detected2?":bool)
              n163 = Get Date/Time In Seconds() -> (seconds since 1Jan1904=w313:timestamp)
              n164 = Format Date/Time String(seconds (now)=w313, UTC format=FALSE) -> (date/time string=→"date/time string":string)  [unwired: 1 in]
              n165 = Compound Arithmetic op=OR(w297, w327) -> (w328:bool)
              n166 = Compound Arithmetic op=OR("Parar la aplicación", "Reset del controlador", "Configuración") -> (w325:bool)
              n167 = xnode "Read/Write Control"("FPGA VI Reference In"=w320, "error in"=w319, "Fotocélula"="Acquire") -> ("FPGA VI Reference Out"=w306:refnum<k20>, "error out"=w305:errorcluster)
              n168 = Compound Arithmetic op=OR("Acquire", w328, w325, w311) -> (w343:bool)
              n169 = Select(t="TEST", s=w328, f="Adquisición") -> (s? t:f=w339:string)
              n170 = Select(t="Configuración", s=w325, f=w339) -> (s? t:f=w316:string)
              "Loop" <- w299
              "Boton Adquirir?" <- "Acquire"
            }
            n171 = call <vilib>:"Watchdog Clear.vi"("error in (no error)"=w278, "watchdogID in"=w279) -> ("error out"=w277:errorcluster)  [unwired: 5 in]
            n172 = xnode "Read/Write Control"("FPGA VI Reference In"=w272, "error in"=w273) -> ("FPGA VI Reference Out"=w271:refnum<k20>, "error out"=w270:errorcluster, "Direccion 0?"=→"Direction 0?":bool)
            n173 = Unbundle By Name(w270) -> ("status"=w290:bool)
            n174 = Select(t="TEST", s=w290, f=w291) -> (s? t:f=w284:string)
            n175 = flat-sequence {
              tunnel: [w294] -> w283
              tunnel: w284 -> [w294]
              frame #0 {
                n176 = Get Date/Time In Seconds() -> (seconds since 1Jan1904=w295:timestamp)
                n177 = To Double Precision Float(number=w295) -> (double precision float=→"Tiempo":dbl)
              }
            }
          }
          frame "Adquisición" {
            n178 = local read "Watchdog config"() -> (w357:T3)
            n179 = call <vilib>:"Watchdog Configure.vi"("error in (no error)"=w356, "expiration actions"=w357, "timeout (1 sec)"=200.0) -> ("error out"=w354:errorcluster, "watchdogID"=w355:u64)  [unwired: 1 in, 2 out]
            n180 = flat-sequence {
              tunnel: w381 -> [w410]
              tunnel: w382 -> [w411]
              tunnel: [w409] -> w371
              tunnel: [w408] -> w370
              tunnel: [w407] -> w369
              tunnel: [w406] -> w368
              tunnel: [w405] -> w367
              tunnel: [w404] -> w366
              tunnel: [w393] -> w359
              tunnel: w355 -> [w392]
              tunnel: w354 -> [w391]
              tunnel: [w392] -> w353
              tunnel: [w391] -> w352
              tunnel: [w427] -> w380
              tunnel: [w444] -> w379
              tunnel: [w443] -> w378
              tunnel: [w442] -> w377
              tunnel: [w435] -> w376
              tunnel: w371 -> [w441]
              tunnel: w370 -> [w440]
              tunnel: w369 -> [w439]
              tunnel: w368 -> [w438]
              tunnel: w367 -> [w437]
              tunnel: w366 -> [w436]
              tunnel: w359 -> [w433]
              tunnel: [w432] -> w358
              tunnel: w353 -> [w431]
              tunnel: w352 -> [w430]
              tunnel: [w428] -> w351
              tunnel: w380 -> [w594]
              tunnel: w379 -> [w589]
              tunnel: w378 -> [w588]
              tunnel: w377 -> [w609]
              tunnel: [w639] -> w363
              tunnel: w376 -> [w641]
              tunnel: [w625] -> w373
              tunnel: [w626] -> w375
              tunnel: [w627] -> w374
              tunnel: w358 -> [w603]
              tunnel: w351 -> [w595]
              tunnel: [w595] -> w349
              tunnel: [w594] -> w348
              frame #0 {
                n181 = local read "Offset_rueda WS 1"() -> (w384:fxp<+/-,24,-4>)
                n182 = local read "Zero channel WS1?"() -> (w395:bool)
                n183 = local read "Offset_rueda WS 2"() -> (w385:fxp<+/-,24,-4>)
                n184 = local read "Count(mSec)"() -> (w394:u32)
                n185 = local read "Zero channel WS2?"() -> (w383:bool)
                n186 = local read "Samples per channel FIFO"() -> (w390:u32)
                n187 = local read "Frecuency rate (Hz)"() -> (w402:dbl)
                n188 = local read "Frecuency rate and CRIO module"() -> (w397:T2)
                n189 = local read "Digital?"() -> (w396:bool)
                n190 = local read "RFID LR6 on?"() -> (w386:bool)
                n191 = xnode "Read/Write Control"("FPGA VI Reference In"=w411, "error in"=w410, "Data Rate"=w397, "Digital?"=w396, "Canal cero WS1?"=w395, "Count(mSec)"=w394, "Offset_WS1"=w384, "Offset_WS2"=w385, "Canal cero WS2?"=w383) -> ("FPGA VI Reference Out"=w401:refnum<k20>, "error out"=w400:errorcluster)
                n192 = case shown="False" w386 {
                  tunnel: [errorcluster {"status"=FALSE, "code"=0, "source"=""} ("error out") w417] -> w393
                  frame False {
                    n193 = local write "TAGs LR6"(string[] []) -> ()
                  }
                  frame True {
                    n194 = local read "RFID_LR6_Error"() -> (w418:errorcluster)
                    n195 = call "LH6HD.vi"("error in (no error)"=w418, "Action"=enum16{"Init", "Start", "Read", "Stop", "Exit"}."Start") -> ("error out"=w417:errorcluster)  [unwired: 8 in, 1 out]
                  }
                }
                n196 = Add(x="Nº inductivos", y="Nº de acelerómetros") -> (x+y=w388:i32)
                n197 = call "DMACalc.vi"("Number of Channels"=w388, "Number of Samples"=w390, "Rate (Hz)"=w402) -> ("Block Size"=w406:u32, "Time to Acquire Block (ms)"=w407:i32, "Host Buffer Size"=w412:u32)  [unwired: 6 in]
                n198 = call "Pathhorafech(SubVI)_varios.vi"("Folder path"=path "c:/Trenes", "Nº de acelerómetros"="Nº de acelerómetros", "Nº inductivos"="Nº inductivos") -> ("Acel_Paths"=w398:path[])  [unwired: 1 in, 1 out]
                "File Name" <- w398
                n199 = for {
                  tunnel: w398 -> [w422] mode=indexing
                  tunnel: [w421] -> w405 mode=indexing
                  tunnel: [w420] -> w404
                  n200 = Open/Create/Replace File(file path (use dialog)=w422, operation (0:open)=T6."replace or create", access (0:read/write)=enum16{"read/write", "read-only", "write-only"}."read/write", disable buffering (F)=TRUE) -> (refnum out=w421:refnum<file>, error out=w420:errorcluster)  [unwired: 1 in, 2 out]
                }
                n201 = xnode "Invoke Method"("FPGA VI Reference In"=w401, "error in"=w400, "Requested Depth"=w412) -> ("FPGA VI Reference Out"=w414:refnum<k20>, "error out"=w413:errorcluster)  [unwired: 1 out]
                n202 = Get Date/Time In Seconds() -> (seconds since 1Jan1904=→"Inicio pasada":timestamp)
                n203 = xnode "Invoke Method"("FPGA VI Reference In"=w414, "error in"=w413) -> ("FPGA VI Reference Out"=w409:refnum<k20>, "error out"=w408:errorcluster)
              }
              frame #1 {
                n204 = while "Data Acquisition" {
                  tunnel: w441 -> [w496]
                  shift-right: [w521] -> _
                  shift-left: u32 0 ("t") -> [w517]
                  tunnel: w439 -> [w522]
                  tunnel: w438 -> [w520]
                  shift-right: [w523] -> w443
                  shift-left: w440 -> [w514]
                  tunnel: [w518] -> w444
                  tunnel: w437 -> [w500]
                  tunnel: [w501] -> w442
                  shift-right: [w499] -> w435
                  shift-left: w436 -> [w510]
                  i -> [w495]
                  stop <- w519 stop-if-true
                  # "Detector de presencia"
                  # "Mide el tiempo de paso del tren y con ello se puede calcular\nla velocidad la unidad"
                  n205 = xnode "Invoke Method"("FPGA VI Reference In"=w496, "error in"=w514, "Number of Elements"=w517, "Timeout (ms)"=0) -> ("FPGA VI Reference Out"=w492:refnum<k20>, "error out"=w498:errorcluster, "Data"=w513:fxp<+/-,24,4>[], "Elements Remaining"=w515:u32)
                  n206 = case "Data Ready" shown="Default" w517 {
                    tunnel: w522 -> [w545 _]
                    tunnel: [w544 u32 0 ("t")] -> w521
                    tunnel: w520 -> [w546 _]
                    tunnel: w515 -> [w543 _]
                    tunnel: w513 -> [_ w568]
                    tunnel: w510 -> [w542 w567]
                    tunnel: [w542 w569] -> w499
                    tunnel: w500 -> [w541 w566]
                    tunnel: [w541 w565] -> w501
                    frame 0 {
                      # "En este caso se compara los elementos que quedan\nen la FIFO del controlador con el tamaño dell bloque\nque aparece en el panel frontal. Si el número de \nelementos en la FIFO es mayor o igual que el tamaño\n del bloque se pasa al siguiente caso y se guardan \nlos datos en un archivo. El reloj que aparece es una\nespera para no consumir recursos."
                      n207 = Greater Or Equal?(x=w543, y=w546) -> (x >= y?=w547:bool)
                      n208 = case shown="False" w547 {
                        tunnel: [u32 0 ("Block Size") w551] -> w544
                        tunnel: [w550 0 ("t")] -> w548
                        tunnel: w545 -> [w550 _]
                        tunnel: w546 -> [_ w551]
                        frame False {
                        }
                        frame True {
                        }
                      }
                      n209 = call "WaitMinTimeBetweenCall.vi"("Minimum ms between calls"=w548) -> ()  [unwired: 2 in]
                    }
                    frame Default {
                      n210 = To Single Precision Float(number=w568) -> (single precision float=w555:sgl[])
                      n211 = Decimate 1D Array(w555) -> (w561:sgl[], w564:sgl[], w563:sgl[], w562:sgl[], w560:sgl[], w559:sgl[], w558:sgl[], w557:sgl[], w556:sgl[], w553:sgl[])
                      n212 = Build Array(w561, w564, w563, w562, w560, w559, w558, w557, w556, w553) -> (w554:sgl[][])
                      n213 = for {
                        tunnel: T7."little-endian" ("byte order (0:big-endian, network order)") -> [w578]
                        shift-right: [w572] -> w569
                        shift-left: w567 -> [w573]
                        tunnel: w554 -> [w576] mode=indexing
                        tunnel: w566 -> [w575] mode=indexing
                        tunnel: [w574] -> w565 mode=indexing
                        n214 = Write to Binary File(file (use dialog)=w575, data=w576, error in=w573, 5:FALSE ("prepend array or string size? (T)"), 9:w578) -> (refnum out=w574:refnum<file>, error out=w572:errorcluster)  [unwired: 2 out]
                      }
                    }
                  }
                  n215 = xnode "Read/Write Control"("FPGA VI Reference In"=w492, "error in"=w498) -> ("FPGA VI Reference Out"=w512:refnum<k20>, "error out"=w511:errorcluster, "Parar"=w488:bool, "Nº Ruedas 1"=→"Nº Wheel 1":i32, "NºRuedas 2"=→"Nº Wheel 2":i32)
                  "Parar" <- w488
                  n216 = case shown="False" w488 {
                    tunnel: [w527 w536] -> w489
                    tunnel: [w529 0.0] -> w504
                    frame False {
                      n217 = local read "Inicio pasada"() -> (w532:timestamp)
                      n218 = Get Date/Time In Seconds() -> (seconds since 1Jan1904=w531:timestamp)
                      n219 = To Double Precision Float(number=w531) -> (double precision float=w530:dbl)
                      n220 = To Double Precision Float(number=w532) -> (double precision float=w533:dbl)
                      n221 = Subtract(x=w530, y=w533) -> (x-y=w529:dbl)
                      "Train pass time (s)" <- w529
                      n222 = local write "Tiempo"(w530) -> ()
                      n223 = local read "Boton Adquirir?"() -> (w524:bool)
                      n224 = Greater?(x=w529, y="Acquisition time") -> (0:w526:bool)
                      n225 = Select(t=w526, s=w524, f=FALSE) -> (s? t:f=w527:bool)
                    }
                    frame True {
                      n226 = local read "Tiempo"() -> (w540:dbl)
                      n227 = Get Date/Time In Seconds() -> (seconds since 1Jan1904=w537:timestamp)
                      n228 = local read "Extra time detection (s)"() -> (w535:dbl)
                      n229 = To Double Precision Float(number=w537) -> (double precision float=w538:dbl)
                      n230 = Subtract(x=w538, y=w540) -> (x-y=w539:dbl)
                      "Acquisition extra time (s)" <- w539
                      n231 = Greater?(x=w539, y=w535) -> (0:w536:bool)
                    }
                  }
                  "Fin" <- w489
                  n232 = local read "Timeout ruedas"() -> (w487:dbl)
                  n233 = xnode ("CheckLate")("FPGA VI Reference In"=w512, "error in"=w511) -> ("FPGA VI Reference Out"=w494:refnum<k20>, "error out"=w507:errorcluster, "Buffer Underflow"=→"Buffer Underflow":bool, "Buffer Overflow"=w497:bool)
                  "Buffer Overflow" <- w497
                  n234 = Greater?(x=w504, y=w487) -> (0:w502:bool)
                  "Timeout ruedas" <- w502
                  n235 = call "ErrorOverFlow.vi"("Buffer Overflow"=w497) -> ("error out"=w505:errorcluster)
                  n236 = call "ErrorUnderFlow.vi"() -> ("error out"=w506:errorcluster)  [unwired: 1 in]
                  n237 = Merge Errors(w507, w506, w505) -> (w493:errorcluster)
                  n238 = Unbundle By Name(w499) -> ("status"=w503:bool)
                  n239 = Unbundle By Name(w493) -> ("status"=w509:bool)
                  n240 = Compound Arithmetic op=OR(w509, w489, w502, w503) -> (w519:bool)
                  "result" <- w519
                  n241 = case "Flush" shown="True" w519 {
                    tunnel: [w579 w584] -> w523
                    tunnel: [w580 w583] -> w518
                    tunnel: w494 -> [w580 w582]
                    tunnel: w493 -> [w579 w581]
                    frame False {
                    }
                    frame True {
                      n242 = xnode "Invoke Method"("FPGA VI Reference In"=w582, "error in"=w581) -> ("FPGA VI Reference Out"=w583:refnum<k20>, "error out"=w584:errorcluster)
                    }
                  }
                  "Block Size" <- w520
                  "Time to Acquire Block (ms)" <- w522
                  "Numeric 3" <- w495
                }
                n243 = call <vilib>:"Watchdog Whack.vi"("error in (no error)"=w430, "reset watchdog after expire? (F)"=TRUE, "watchdogID in"=w431) -> ("error out"=w427:errorcluster, "watchdogID out"=w428:u64)  [unwired: 2 in, 1 out]
                n244 = local read "RFID LR6 on?"() -> (w426:bool)
                n245 = case shown="True" w426 {
                  tunnel: w433 -> [w445 w451]
                  tunnel: [w445 w450] -> w432
                  frame False {
                  }
                  frame True {
                    n246 = while {
                      shift-right: [w458] -> w450
                      shift-left: w451 -> [w459]
                      shift-right: [w457] -> w448
                      shift-left: string[] [] -> [w456]
                      shift-right: [w452] -> w446
                      shift-left: i32[] [] -> [w453]
                      i -> [w454]
                      stop <- w455 stop-if-true
                      n247 = case shown="No Error" w459 {
                        selector: w459 -> [w470 _]
                        tunnel: [w469 w485] -> w458
                        tunnel: [w465 string[] []] -> w457
                        tunnel: w456 -> [w464 _]
                        tunnel: w454 -> [w463 _]
                        tunnel: w453 -> [w462 _]
                        tunnel: [w461 i32[] []] -> w452
                        frame No Error {
                          n248 = call "LH6HD.vi"("error in (no error)"=w470, "Action"=enum16{"Init", "Start", "Read", "Stop", "Exit"}."Read") -> ("error out"=w469:errorcluster, "Tag"=w466:string)  [unwired: 8 in]
                          n249 = Not Equal?(x="", y=w466) -> (x != y?=w467:bool)
                          n250 = case shown="False" w467 {
                            tunnel: w466 -> [_ w479]
                            tunnel: [w473 w478] -> w465
                            tunnel: w464 -> [w473 w477]
                            tunnel: w463 -> [_ w474]
                            tunnel: w462 -> [w472 w476]
                            tunnel: [w472 w475] -> w461
                            frame False {
                            }
                            frame True {
                              n251 = Build Array (concatenate)(w477, w479) -> (w478:string[])
                              n252 = Build Array (concatenate)(w476, w474) -> (w475:i32[])
                            }
                          }
                        }
                        frame Error {
                          n253 = local read "LR6 IP address"() -> (w482:string)
                          n254 = local read "DeviceAddress"() -> (w480:u8)
                          n255 = local read "Port LR6"() -> (w483:u16)
                          n256 = call "LH6HD.vi"("DeviceAddress"=w480, "Reader Port"=w483, "IP Address"=w482, "Action"=enum16{"Init", "Start", "Read", "Stop", "Exit"}."Init") -> ("error out"=w485:errorcluster)  [unwired: 6 in, 1 out]
                        }
                      }
                      n257 = Wait Until Next ms Multiple(millisecond multiple=u32 500) -> ()  [unwired: 1 out]
                      n258 = local read "result"() -> (w455:bool)
                      "it-LR6" <- w454
                    }
                    "TAGs LR6" <- w448
                    "it-read-LR6" <- w446
                  }
                }
              }
              frame #2 {
                n259 = local read "RFID LR6 on?"() -> (w590:bool)
                n260 = local read "AURA wheel test"() -> (w586:bool)
                n261 = case shown="False" w586 {
                  tunnel: [w649 string[] ["A0000000000000000TESTNEM7", "A0000000000000000TESTNEM8"]] -> w585
                  frame False {
                    n262 = local read "TAGs LR6"() -> (w649:string[])
                  }
                  frame True {
                  }
                }
                n263 = Array Size(array=w609) -> (size(s)=w607:i32)
                n264 = local read "timeout ms (60000)"() -> (w593:i32)
                n265 = local read "bytes to read"() -> (w592:i32)
                n266 = local read "RFID NEM on?"() -> (w591:bool)
                n267 = Decrement(x=w607) -> (x-1=w608:i32)
                n268 = case shown="False" w590 {
                  tunnel: w603 -> [w651 w653]
                  tunnel: [w651 w652] -> w602
                  frame False {
                  }
                  frame True {
                    n269 = call "LH6HD.vi"("error in (no error)"=w653, "Action"=enum16{"Init", "Start", "Read", "Stop", "Exit"}."Stop") -> ("error out"=w652:errorcluster)  [unwired: 8 in, 1 out]
                  }
                }
                n270 = local read "RFID Port"() -> (w624:u16)
                n271 = local read "RFID Error"() -> (w635:errorcluster)
                n272 = local read "RFID IP"() -> (w606:string)
                n273 = local read "RFID_ID"() -> (w634:refnum<k5>)
                n274 = Index Array(array=w609, index=w608) -> (element=w617:refnum<file>)
                n275 = local write "result"(FALSE ("result")) -> ()
                n276 = case shown="True" w591 {
                  tunnel: [_ w666] -> w636
                  tunnel: w635 -> [w656 w665]
                  tunnel: w634 -> [w655 w664]
                  tunnel: [w655 w663] -> w633
                  tunnel: [w656 w662] -> w628
                  tunnel: w624 -> [_ w661]
                  tunnel: w606 -> [_ w660]
                  tunnel: [_ w659] -> w587
                  tunnel: w593 -> [_ w658]
                  tunnel: w592 -> [_ w657]
                  frame False {
                  }
                  frame True {
                    n277 = call "RFID_28_03_12.vi"("BYTES TO READ"=w657, "TIMEOUT"=w658, "RFID_Error"=w665, "Puerto RFID"=w661, "IP RFID"=w660, "RFID ID"=w664) -> ("RFID Error"=w662:errorcluster, "connection ID out"=w663:refnum<k5>, "TAGs HEX"=w659:string[], "Unidad"=w666:u32)  [unwired: 1 in]
                  }
                }
                "TAGs HEX" <- w587
                n278 = local write "RFID_LR6_Error"(w602) -> ()
                n279 = for {
                  tunnel: w585 -> [w669] mode=indexing
                  tunnel: [w667] -> w596 mode=indexing
                  n280 = Search and Replace String(input string=w669, search string="00") -> (result string=w667:string)  [unwired: 6 in, 3 out]
                }
                n281 = xnode "Read/Write Control"("FPGA VI Reference In"=w589, "error in"=w588) -> ("FPGA VI Reference Out"=w638:refnum<k20>, "error out"=w637:errorcluster, "Chassis Temperature"=w647:i16)
                n282 = Index Array(array=w587) -> (element=w601:string)  [unwired: 1 in]
                n283 = Not Equal?(x=w601, y="" ("delimiter (\\t)")) -> (x != y?=w599:bool)
                "Plataformas?" <- w599
                n284 = case shown="True" w599 {
                  tunnel: w596 -> [w670 w671]
                  tunnel: [w670 w673] -> w604
                  tunnel: w587 -> [_ w672]
                  frame False {
                  }
                  frame True {
                    n285 = call "Union_TAGs_RFIDs.vi"("TAGs LR6"=w671, "TAGs HEX"=w672) -> ("TAGs"=w673:string[])
                  }
                }
                "TAGs" <- w604
                n286 = Divide(x=w647, y=4.0) -> (x/y=w648:dbl)
                "Temperature (ºC)" <- w648
                n287 = local read "Train pass time (s)"() -> (w631:dbl)
                n288 = local read "File Name"() -> (w616:path[])
                n289 = Multiply(x=w631, y=1000.0) -> (x*y=w629:dbl)
                n290 = for {
                  shift-right: [w679] -> w622
                  shift-left: string[] [] -> [w678]
                  tunnel: w604 -> [w677] mode=indexing
                  n291 = Insert Into Array(array=w678, new element=w677) -> (w679:string[])  [unwired: 1 in]
                }
                n292 = Build Array(w648, w629, w636) -> (w642:dbl[])
                n293 = local write "RFID_ID"(w633) -> ()
                n294 = local write "RFID Error"(w628) -> ()
                n295 = Delete From Array(array=w616) -> (deleted portion=w615:path)  [unwired: 2 in, 1 out]
                n296 = To Single Precision Float(number=w642) -> (single precision float=w645:sgl[])
                n297 = xnode "Read/Write Control"("FPGA VI Reference In"=w638, "error in"=w637, "Stop"=TRUE ("stop")) -> ("FPGA VI Reference Out"=w619:refnum<k20>, "error out"=w618:errorcluster)
                n298 = Path To String(path=w615) -> (string=w621:string)
                n299 = Write to Binary File(file (use dialog)=w617, data=w645, error in=w641, 5:FALSE ("prepend array or string size? (T)"), 9:T7."little-endian" ("byte order (0:big-endian, network order)")) -> (error out=w614:errorcluster)  [unwired: 3 out]
                n300 = local read "Timeout ruedas"() -> (w632:bool)
                n301 = Build Array (concatenate)(w621, w622) -> (w597:string[])
                n302 = local read "TAGS leidos"() -> (w610:path)
                n303 = for {
                  shift-right: [w676] -> w625
                  shift-left: w614 -> [w675]
                  tunnel: w609 -> [w674] mode=indexing
                  n304 = Close File(refnum=w674, error in=w675) -> (error out=w676:errorcluster)  [unwired: 1 out]
                }
                n305 = xnode "Invoke Method"("FPGA VI Reference In"=w619, "error in"=w618) -> ("FPGA VI Reference Out"=w627:refnum<k20>, "error out"=w626:errorcluster)
                n306 = call-poly <vilib>:"Write Delimited Spreadsheet.vi"("file path (dialog if empty)"=w610, "1D data"=w597, "append to file? (new file:F)"=TRUE ("transpose? (no:F)"), "transpose? (no:F)"=TRUE ("append to file? (new file:F)"), "delimiter (\\t)"=";" ("delimiter (\\t)")) -> ()  [unwired: 9 in, 2 out]
                n307 = Select(t="TEST", s=w632, f="Procesado") -> (s? t:f=w639:string)
              }
            }
            n308 = call <vilib>:"Watchdog Clear.vi"("error in (no error)"=w348, "watchdogID in"=w349) -> ("error out"=w350:errorcluster)  [unwired: 5 in]
            n309 = Unbundle By Name(w375) -> ("status"=w364:bool)
            n310 = Unbundle By Name(w373) -> ("status"=w365:bool)
            n311 = Merge Errors(w373, w350) -> (w372:errorcluster)
            n312 = Compound Arithmetic op=OR(w364, w365) -> (w362:bool)
            n313 = Select(t="TEST", s=w362, f=w363) -> (s? t:f=w360:string)
          }
          frame "Procesado" {
            n314 = local read "Watchdog config"() -> (w686:T3)
            n315 = call <vilib>:"Watchdog Configure.vi"("error in (no error)"=w689, "expiration actions"=w686, "timeout (1 sec)"=300.0) -> ("error out"=w688:errorcluster, "watchdogID"=w685:u64)  [unwired: 1 in, 2 out]
            n316 = flat-sequence {
              tunnel: w688 -> [w711]
              tunnel: [w714] -> w691
              tunnel: w685 -> [w706]
              tunnel: [w705] -> w684
              tunnel: [w704] -> w683
              tunnel: [w925] -> w701
              tunnel: w691 -> [w925]
              tunnel: [w919] -> w682
              tunnel: w684 -> [w919]
              tunnel: [w918] -> w681
              tunnel: w683 -> [w918]
              frame #0 {
                n317 = flat-sequence {
                  tunnel: [w784] -> w713
                  tunnel: [w769] -> w712
                  tunnel: w711 -> [w735]
                  tunnel: [w772] -> w710
                  tunnel: [w760] -> w707
                  tunnel: [w771] -> w709
                  tunnel: [w759] -> w708
                  tunnel: w706 -> [w736]
                  tunnel: [w733] -> w705
                  tunnel: [w732] -> w704
                  frame #0 {
                    # "No es necesario leer el segundo archivo"
                    # "Distancia de\nla unidad"
                    n318 = local read "Tabla_flota"() -> (w768:string[][])
                    n319 = case shown="True" "AURA wheel test" {
                      tunnel: [w788 path[] [path "c:/Trenes_prueba/A_0_TEST.bin", path "c:/Trenes_prueba/A_1_TEST.bin", path "c:/Trenes_prueba/A_2_TEST.bin", path "c:/Trenes_prueba/A_3_TEST.bin", path "c:/Trenes_prueba/A_4_TEST.bin", path "c:/Trenes_prueba/A_5_TEST.bin", path "c:/Trenes_prueba/A_6_TEST.bin", path "c:/Trenes_prueba/A_7_TEST.bin", path "c:/Trenes_prueba/I_0_TEST.bin", path "c:/Trenes_prueba/I_1_TEST.bin"]] -> w728
                      tunnel: [w787 w789] -> w716
                      frame False {
                        n320 = local read "TAGs"() -> (w787:string[])
                        n321 = local read "File Name"() -> (w788:path[])
                      }
                      frame True {
                        w789 = string[] ["A0000000000000000TESTNEM7", "A0000000000000000TESTNEM8"]
                        n322 = local write "TAGs LR6"(w789) -> ()
                      }
                    }
                    n323 = call <vilib>:"Watchdog Whack.vi"("error in (no error)"=w735, "reset watchdog after expire? (F)"=TRUE, "watchdogID in"=w736) -> ("error out"=w732:errorcluster, "watchdogID out"=w733:u64)  [unwired: 2 in, 1 out]
                    n324 = call "Series_ejes_flota.vi"("Tabla_flota"=w768, "Tags"=w716) -> ("Nº Ejes"=w727:i32[], "Series del convoy"=w762:string[])  [unwired: 2 in, 1 out]
                    "Nº Ejes" <- w727
                    n325 = local read "Puntos medios de las ventanas"() -> (w770:dbl[][])
                    n326 = Array Size(array=w728) -> (size(s)=w778:i32)
                    n327 = Add Array Elements(numeric array=w727) -> (sum=w731:i32)
                    "Train axles" <- w731
                    n328 = Subtract(x=w778, y=2 ("length")) -> (x-y=w780:i32)
                    n329 = Array Size(array=w762) -> (size(s)=→"Nº UTs":i32)
                    n330 = Delete From Array(array=w728, length=2, index=w780) -> (deleted portion=w749:path[], array with subset deleted=w771:path[])
                    n331 = Index Array(array=w749) -> (element #1=w729:path, element #2=w730:path)  [unwired: 2 in]
                    n332 = Read from Binary File(5:sgl 0.0, 9:T7."little-endian" ("byte order (0:big-endian, network order)"), 10:-1 ("count (1)"), 11:w730) -> (0:w776:errorcluster, 2:w751:sgl[], 3:w777:refnum<file>)  [unwired: 1 in, 2 out]
                    n333 = local read "Frecuency rate (Hz)"() -> (w718:dbl)
                    n334 = local read "Series_flota"() -> (w767:string[])
                    n335 = local read "Offset_rueda WS 2"() -> (w719:fxp<+/-,24,-4>)
                    n336 = Close File(refnum=w777, error in=w776) -> (error out=w772:errorcluster)  [unwired: 1 out]
                    n337 = Read from Binary File(5:sgl 0.0, 9:T7."little-endian" ("byte order (0:big-endian, network order)"), 10:-1 ("count (1)"), 11:w729) -> (0:w747:errorcluster, 2:w739:sgl[], 3:w748:refnum<file>)  [unwired: 1 in, 2 out]
                    n338 = Array Size(array=w751) -> (size(s)=w766:i32)
                    n339 = Close File(refnum=w748, error in=w747) -> ()  [unwired: 2 out]
                    n340 = Subtract(x=w766, y=3 ("length")) -> (x-y=w764:i32)
                    n341 = Array Size(array=w739) -> (size(s)=w743:i32)
                    n342 = Delete From Array(array=w751, length=3, index=w764) -> (array with subset deleted=w725:sgl[])  [unwired: 1 out]
                    n343 = call "Distancias_ejes_convoy.vi"("Series_flota1"=w762, "Ejes_UT"=w727, "Puntos medios de las ventanas"=w770, "Series_flota"=w767) -> ("Distancias_entre_ejes_convoy"=w769:dbl[])  [unwired: 1 in]
                    n344 = Subtract(x=w743, y=3 ("length")) -> (x-y=w741:i32)
                    n345 = Delete From Array(array=w739, length=3, index=w741) -> (array with subset deleted=w738:sgl[])  [unwired: 1 out]
                    n346 = call "Analogico_digital.vi"("Array"=w725, "Offset WS"=w719, "Frecuencia muestreo"=w718) -> ("array w/ subset deleted"=w720:sgl[], "Tiempo\npaso"=w717:dbl)  [unwired: 6 in]
                    "Digital wheels" <- w720
                    n347 = call "Puntos medio de pulso.vi"("DI Inductivo"=w720) -> ("Puntos"=w784:sgl[], "Número de ejes"=w752:i32)  [unwired: 1 in]
                    "Detected axles" <- w752
                    n348 = Build Array(w725, w738) -> (→"Current Wheel sensor":sgl[][])
                    n349 = local read "it-LR6"() -> (w755:i32)
                    n350 = local read "it-read-LR6"() -> (w756:i32[])
                    n351 = local read "Plataformas?"() -> (w754:bool)
                    n352 = local read "TAGs"() -> (w758:string[])
                    n353 = local read "TAGs LR6"() -> (w757:string[])
                    n354 = Decrement(x=w752) -> (x-1=w783:i32)
                    n355 = disable-structure shown="Enabled" {
                      disable-tunnel: w725 -> [w797 w800]
                      disable-tunnel: [FALSE ("element") TRUE ("element")] -> w722
                      disable-tunnel: [w791 w799] -> w721
                      frame Disabled {
                        n356 = Equal?(x=w797, y=0.0) -> (x = y?=w794:bool[])
                        n357 = Equal?(x=w797, y=1.0) -> (x = y?=w795:bool[])
                        n358 = Or(x=w794, y=w795) -> (x .or. y?=w791:bool[])
                      }
                      frame Enabled {
                        n359 = Greater?(x=w800, y=0.1) -> (0:w799:bool[])
                      }
                    }
                    n360 = call "Calculo_Velocidad.vi"("Tiempo de paso (s)"=w717, "Ejes"=w783, "Puntos iniciales de las ventanas"=w769) -> ("V (m/s)"=→"V (m/s)":dbl, "Longitud de la unidad"=→"Longitud de la unidad":dbl)
                    n361 = call "TAGs_AURAwheel.vi"("Nº Ejes"=w727, "TAGs"=w758, "Ejes_convoy"=w731, "it-LR6"=w755, "TAGs LR6"=w757, "it-read-LR6"=w756, "Plataformas?"=w754) -> ("TAGS_AURA"=→"TAGs_AURAwheel":string[][])  [unwired: 1 in]
                    n362 = Get Volume Info(11:path "c:/" ("path")) -> (1:→"Hard drive status (bytes)":i64)  [unwired: 1 in, 5 out]
                    n363 = Equal?(x=w731, y=w752) -> (x = y?=w759:bool)
                    n364 = Search 1D Array(1D array=w721, element=w722) -> (index of element=w723:i32)  [unwired: 1 in]
                    n365 = Equal?(x=w723, y=-1) -> (x = y?=w726:bool)
                    n366 = And(x=w759, y=w726) -> (x .and. y?=w760:bool)
                    "Valid \nfile?" <- w760
                  }
                }
                n367 = case shown="True" w707 {
                  tunnel: w710 -> [w804 w835]
                  tunnel: [w804 w834] -> w714
                  tunnel: w713 -> [_ w839]
                  tunnel: w712 -> [_ w837]
                  tunnel: w709 -> [_ w838]
                  tunnel: w708 -> [w802 _]
                  frame False {
                    n368 = local read "File Name"() -> (w803:path[])
                    n369 = for {
                      tunnel: w803 -> [w806] mode=indexing
                      tunnel: w802 -> [w805]
                      n370 = flat-sequence {
                        tunnel: w806 -> [w816]
                        tunnel: [w816] -> w809
                        tunnel: [w815] -> w808
                        tunnel: w805 -> [w814]
                        tunnel: w809 -> [w823]
                        tunnel: [w822] -> w807
                        tunnel: w808 -> [w822]
                        tunnel: w807 -> [w825]
                        frame #0 {
                          w815 = path "c:/Est_Adq.csv" ("file path (use dialog)")
                          n371 = Path To String(path=w816) -> (string=w817:string)
                          n372 = Select(t="Nº Ejes detectados WS diferente a Nº Ejes TAGs" ("delimiter (\\t)"), s=w814, f="La señal del inductivo no es digital" ("delimiter (\\t)")) -> (s? t:f=w811:string)
                          n373 = Build Array(w817, w811) -> (w810:string[])
                          n374 = call-poly <vilib>:"Write Delimited Spreadsheet.vi"("file path (dialog if empty)"=w815, "1D data"=w810, "append to file? (new file:F)"=FALSE ("transpose? (no:F)"), "transpose? (no:F)"=TRUE ("append to file? (new file:F)"), "delimiter (\\t)"=";" ("delimiter (\\t)")) -> ()  [unwired: 9 in, 2 out]
                        }
                        frame #1 {
                          n375 = local read "Borrar archivos\nadquisicion con error"() -> (w821:bool)
                          n376 = case shown="True" w821 {
                            tunnel: w823 -> [_ w824]
                            frame False {
                            }
                            frame True {
                              n377 = Delete(path (use dialog)=w824) -> ()  [unwired: 1 in, 6 out]
                            }
                          }
                        }
                        frame #2 {
                          n378 = File/Directory Info(path=w825) -> (size=w828:i64)  [unwired: 1 in, 6 out]
                          n379 = Greater?(x=w828, y=i64 1000000) -> (0:w826:bool)
                          n380 = case shown="True" w826 {
                            tunnel: w825 -> [_ w829]
                            frame False {
                            }
                            frame True {
                              n381 = Delete(path (use dialog)=w829) -> ()  [unwired: 4 in, 3 out]
                            }
                          }
                        }
                      }
                    }
                  }
                  frame True {
                    n382 = flat-sequence {
                      tunnel: w839 -> [w909]
                      tunnel: w838 -> [w906]
                      tunnel: w837 -> [w910]
                      tunnel: [w894] -> w836
                      frame #0 {
                        # "SALIDA \n\nMáximos por rueda inductivo"
                        # "8 acelerómetros"
                        # "Velocidad"
                        n383 = local read "Distancia de acelerómetros"() -> (w898:dbl[])
                        n384 = local read "Parámetros acelerómetros"() -> (w905:dbl[])
                        n385 = local read "Frecuency rate (Hz)"() -> (w908:dbl)
                        n386 = local read "Distancias generales"() -> (w903:dbl[])
                        n387 = local read "dt RMS"() -> (w907:dbl)
                        n388 = local read "Detected axles"() -> (w904:i32)
                        n389 = local read "Direction 0?"() -> (w895:bool)
                        n390 = Index Array(array=w903, index=1) -> (element=w901:dbl)
                        n391 = Select(t=0.0, s=w895, f=w901) -> (s? t:f=w899:dbl)
                        n392 = Subtract(x=w899, y=w898) -> (x-y=w897:dbl[])
                        n393 = Absolute Value(x=w897) -> (abs(x)=w896:dbl[])
                        n394 = call "Procesado_aRMS_BIdirecc.vi"("Paths_canales_aRMS"=w906, "Ejes Procesados"=w904, "Distancias\nacelerometros"=w896, "Distancias generales (m)"=w903, "Distancias centrales de las ruedas\n               configuración (m)"=w910, "Frecuencia de muestreo"=w908, "Parámetros acelerómetros"=w905, "dt RMS 2"=w907, "Puntos"=w909) -> ("Max RMS Ruedas"=w893:dbl[][])  [unwired: 2 in]
                        n395 = Transpose 2D Array(2D array=w893) -> (transposed array=w894:dbl[][])
                        "Max Wheel RMS" <- w894
                      }
                    }
                    n396 = local read "Use Aura?"() -> (w833:bool)
                    n397 = local read "TAGs_AURAwheel"() -> (w831:string[][])
                    n398 = local read "Nº Ejes"() -> (w830:i32[])
                    n399 = for {
                      tunnel: w833 -> [w844]
                      tunnel: [w843] -> w832 mode=indexing
                      tunnel: w831 -> [w842] mode=indexing
                      shift-right: [w841] -> _
                      shift-left: w836 -> [w845]
                      tunnel: w830 -> [w840] mode=indexing
                      # "dev.api.aurawheel.com"
                      n400 = case shown="True" w844 {
                        tunnel: w845 -> [w846 w858]
                        tunnel: [errorcluster {"status"=FALSE, "code"=0, "source"=""} ("error out") w863] -> w843
                        tunnel: w842 -> [_ w859]
                        tunnel: [w846 w857] -> w841
                        tunnel: w840 -> [_ w855]
                        frame False {
                        }
                        frame True {
                          w867 = cluster{"status":string} {"status"=""}
                          n401 = local read "Parametros AuraWheel"() -> (w892:string[])
                          n402 = Delete From Array(array=w858, length=w855, index (row)=0) -> (deleted portion=w854:dbl[][], array with subset deleted=w857:dbl[][])  [unwired: 1 in]
                          n403 = Get Date/Time In Seconds() -> (seconds since 1Jan1904=w888:timestamp)
                          n404 = Format Date/Time String(time format string (%c)="%H:%M:%S%3u", seconds (now)=w888) -> (date/time string=w886:string)  [unwired: 1 in]
                          n405 = Get Date/Time In Seconds() -> (seconds since 1Jan1904=w862:timestamp)
                          n406 = Scan From String(format string="%d:%d:%f", input string=w886) -> (output 1=w883:i32, output 2=w882:i32, output 3=w880:dbl)  [unwired: 5 in, 3 out]
                          n407 = local read "V (m/s)"() -> (w850:dbl)
                          n408 = local read "Temperature (ºC)"() -> (w860:dbl)
                          n409 = Multiply(x=w850, y=3.6) -> (x*y=w848:dbl)
                          n410 = Multiply(x=w880, y=1000.0) -> (x*y=w876:dbl)
                          n411 = call "Time_to_ms.vi"("seconds since 1Jan1904"=w862) -> ("Numeric"=w861:dbl)  [unwired: 1 in]
                          n412 = Multiply(x=w882, y=60000) -> (x*y=w877:i32)
                          n413 = Multiply(x=3600000, y=w883) -> (x*y=w878:i32)
                          n414 = Index Array(array=w892) -> (element #1=w853:string, element #2=w852:string, element #3=w851:string)  [unwired: 3 in]
                          n415 = call "aw_WRDCluster_8acel.vi"("Array TAGs"=w859, "Max RMS Ruedas"=w854, "TimeStamp"=w861, "p_sp"=w848, "p_tp"=w860) -> ("JSON cluster"=w889:T9)  [unwired: 1 in]
                          n416 = Compound Arithmetic op=ADD(w878, w877, w876) -> (w875:dbl)
                          n417 = To Variant(anything=w889) -> (Variant=w872:variant)
                          n418 = To Unsigned Long Integer(number=w875) -> (unsigned 32bit integer=w874:u32)
                          n419 = call "gjson_Create.vi"("JSON Object in"=w872) -> ("error out"=w870:errorcluster, "JSON String Out"=w871:string)  [unwired: 9 in]
                          n420 = Number To Decimal String(number=w874) -> (decimal integer string=w873:string)  [unwired: 1 in]
                          n421 = To Variant(anything=w867) -> (Variant=w866:variant)
                          n422 = call "aw_SendData.vi"("pwd"=w853, "x-nem-datetime"=w873, "User"=w852, "error in"=w870, "JSON Object"=w871, "URL"=w851) -> ("error out"=w868:errorcluster, "Response JSON"=w869:string, "Response headers"=→"Response headers":string)  [unwired: 3 in]
                          n423 = call "gjson_Parse.vi"("error in"=w868, "JSON String In"=w869, "JSON Cluster"=w866) -> ("error out"=w864:errorcluster, "JSON Cluster Out"=w865:variant)  [unwired: 7 in]
                          n424 = Variant To Data(error in=w864, type=w867, Variant=w865) -> (data=→"data":cluster{"status":string}, error out=w863:errorcluster)
                          "AURA error" <- w863
                        }
                      }
                    }
                    n425 = Merge Errors(w832, w835) -> (w834:errorcluster)
                  }
                }
              }
              frame #1 {
                n426 = local read "Bytes libre despues de borrar"() -> (w915:u32)
                n427 = local read "Borrar archivos\nadquisicion con error"() -> (w911:bool)
                n428 = local read "Valid \nfile?"() -> (w914:bool)
                n429 = local read "Bytes min libre"() -> (w916:u32)
                n430 = local read "Max archivos"() -> (w917:u32)
                n431 = local read "TAGS leidos"() -> (w921:path)
                n432 = Not(x=w911) -> (.not. x?=w912:bool)
                n433 = File/Directory Info(path=w921) -> (size=w924:i64)  [unwired: 1 in, 6 out]
                n434 = local read "Path TEST"() -> (w920:path)
                n435 = Or(x=w914, y=w912) -> (x .or. y?=w913:bool)
                n436 = Greater?(x=w924, y=i64 1000000) -> (0:w922:bool)
                n437 = case shown="True" w913 {
                  frame False {
                  }
                  frame True {
                    n438 = local read "File Name"() -> (w927:path[])
                    n439 = call "Comprimir_a_1_archivo.vi"("Acel_paths"=w927) -> ("path_Pasada"=→"created path":path)
                  }
                }
                n440 = case shown="True" w922 {
                  tunnel: w921 -> [_ w928]
                  frame False {
                  }
                  frame True {
                    n441 = Delete(path (use dialog)=w928) -> ()  [unwired: 4 in, 3 out]
                  }
                }
                n442 = call "BORRADO_MEJORADO_Gonzalo.vi"("Bytes LIBRE OK"=w915, "Bytes Minimo de Memoria libre"=w916) -> ()  [unwired: 10 in]
                n443 = call "Borrar_carpeta.vi"("Nº Archivos Max"=w917, "Path Carpeta"=w920) -> ()  [unwired: 1 in]
              }
            }
            n444 = call <vilib>:"Watchdog Clear.vi"("error in (no error)"=w681, "watchdogID in"=w682) -> ("error out"=w680:errorcluster)  [unwired: 5 in]
            n445 = local read "RFID Error"() -> (w692:errorcluster)
            n446 = Merge Errors(w701, w680) -> (w693:errorcluster)
            n447 = Merge Errors(w690, w692, w693) -> (w702:errorcluster)
            n448 = Unbundle By Name(w702) -> ("status"=w696:bool)
            n449 = Select(t="Descarga datos", s=FALSE, f="Espera") -> (s? t:f=w698:string)
            n450 = Select(t="TEST", s=w696, f=w698) -> (s? t:f=w695:string)
          }
          frame "TEST" {
            n451 = local read "Watchdog config"() -> (w937:T3)
            n452 = call <vilib>:"Watchdog Configure.vi"("expiration actions"=w937, "timeout (1 sec)"=200.0) -> ("error out"=w938:errorcluster, "watchdogID"=w935:u64)  [unwired: 2 in, 2 out]
            n453 = flat-sequence {
              tunnel: [w953] -> w942
              tunnel: w938 -> [w948]
              tunnel: w940 -> [w967]
              tunnel: [w966] -> w930
              tunnel: [w949] -> w939
              tunnel: w935 -> [w947]
              tunnel: [w946] -> w933
              tunnel: w934 -> [w945]
              tunnel: [w944] -> w932
              frame #0 {
                n454 = call <vilib>:"Watchdog Whack.vi"("error in (no error)"=w948, "reset watchdog after expire? (F)"=TRUE, "watchdogID in"=w947) -> ("error out"=w944:errorcluster, "watchdogID out"=w946:u64)  [unwired: 2 in, 1 out]
                n455 = Get Date/Time In Seconds() -> (seconds since 1Jan1904=w960:timestamp)
                n456 = local read "Ultimo TEST"() -> (w961:timestamp)
                n457 = To Double Precision Float(number=w960) -> (double precision float=w962:dbl)
                n458 = Subtract(x=w962, y=3600.0) -> (x-y=w964:dbl)
                n459 = To Time Stamp(1:w964) -> (0:w965:timestamp)
                n460 = In Range and Coerce(upper limit=w960, x=w961, lower limit=w965) -> (In Range?=w959:bool)  [unwired: 1 out]
                n461 = case shown="False" w959 {
                  tunnel: w945 -> [w996 _]
                  tunnel: w967 -> [w972 w1011]
                  tunnel: [w981 errorcluster {"status"=FALSE, "code"=0, "source"=""} ("error out")] -> w966
                  tunnel: [w972 w1011] -> w949
                  frame False {
                    n462 = local read "Timeout ruedas"() -> (w973:bool)
                    n463 = local read "Aviso no detección"() -> (w979:string)
                    n464 = local read "Aviso temperatura"() -> (w978:string)
                    n465 = case shown="True" w973 {
                      selector: w973 -> [_ w1008]
                      tunnel: ["\r" w1009] -> w971
                      frame False {
                      }
                      frame True {
                        w998 = "\n"
                        n466 = local read "Nº Wheel 1"() -> (w1005:i32)
                        n467 = local read "Nº Wheel 2"() -> (w1000:i32)
                        n468 = call "ErrorRuedas.vi"("Buffer Overflow"=w1008) -> ("error out"=w1010:errorcluster)
                        n469 = Number To Decimal String(number=w1005) -> (decimal integer string=w1003:string)  [unwired: 1 in]
                        n470 = Number To Decimal String(number=w1000) -> (decimal integer string=w999:string)  [unwired: 1 in]
                        n471 = Concatenate Strings("Error Wheel sensors", "\n", "WS1 (ruedas):", w1003, w998, "WS2 (ruedas):", w999, w998) -> (w1001:string)
                        n472 = call "Error.vi"("Error con..."=w1001, "error comunicacion 2"=w1010) -> ("String"=w1009:string)
                      }
                    }
                    n473 = local read "RFID Error"() -> (w975:errorcluster)
                    n474 = local read "RFID_LR6_Error"() -> (w969:errorcluster)
                    n475 = local read "DC OK"() -> (w977:string)
                    n476 = call "Cabecera.vi"() -> ("String"=w994:string)
                    n477 = call "Adquisicion.vi"("Aviso no detección"=w979) -> ("String"=w993:string)
                    n478 = call "Temperatura.vi"("Aviso temperatura"=w978) -> ("String"=w992:string)
                    n479 = call "Fuente.vi"("DC OK"=w977) -> ("String"=w991:string)
                    n480 = call "FPGA.vi"("error out"=w972) -> ("String"=w990:string)
                    n481 = call "Escritura.vi"("error out"=w996) -> ("String"=w989:string)
                    n482 = call "Error.vi"("Error con..."="Error con el lecto RFID NEM", "error comunicacion 2"=w975) -> ("String"=w974:string)
                    n483 = call "Error.vi"("Error con..."="Error con el lecto RFID LR6-HD", "error comunicacion 2"=w969) -> ("String"=w968:string)
                    n484 = Concatenate Strings(w994, w993, w992, w991, w990, w989, w974, w968, w971) -> (w995:string)
                    n485 = call "STRINGhorafechA(SubVI).vi"() -> ("STRINGhora_fecha"=w988:string)
                    n486 = Concatenate Strings(w988, ".txt" ("string")) -> (w984:string)
                    n487 = Get Date/Time In Seconds() -> (seconds since 1Jan1904=→"Ultimo TEST":timestamp)
                    n488 = Build Array("c", "TEST" ("element"), w984) -> (w986:string[])
                    n489 = Array of Strings to Path(0:w986) -> (2:w982:path)  [unwired: 1 out]
                    n490 = Write to Text File(file (use dialog)=w982, text=w995) -> (error out=w981:errorcluster)  [unwired: 1 in, 3 out]
                  }
                  frame True {
                  }
                }
                n491 = local read "Fallo fotocelula"() -> (w952:bool)
                n492 = Unbundle By Name(w949) -> ("status"=w950:bool)
                n493 = local read "T fuera rango"() -> (w958:bool)
                n494 = Compound Arithmetic op=OR(w950, w952) -> (w951:bool)
                n495 = local write "Reset del controlador"(w951) -> ()
                n496 = Select(t="Escape", s=w958, f="Espera") -> (s? t:f=w955:string)
                n497 = Select(t="Configuracion", s=w951, f=w955) -> (s? t:f=w953:string)
              }
            }
            n498 = call <vilib>:"Watchdog Clear.vi"("error in (no error)"=w932, "watchdogID in"=w933) -> ("error out"=w931:errorcluster)  [unwired: 5 in]
            n499 = Merge Errors(w931, w930) -> (w929:errorcluster)
          }
        }
        "Status" <- w77
        "Write/read error" <- w79
        n500 = local read "Parar la aplicación"() -> (w76:bool)
      }
      n501 = xnode "Close FPGA VI Reference"("FPGA VI Reference In"=w69, "error in"=w68) -> ("error out"=→"FPGA error":errorcluster)
    }
    frame #3 {
      n502 = local read "RFID_ID"() -> (w1015:refnum<k5>)
      n503 = call "LH6HD.vi"("Action"=enum16{"Init", "Start", "Read", "Stop", "Exit"}."Stop") -> ("error out"=→"RFID_LR6_Error":errorcluster)  [unwired: 9 in, 1 out]
      n504 = TCP Close Connection(connection ID=w1015) -> (error out=→"RFID Error":errorcluster)  [unwired: 1 in, 2 out]
    }
  }
